vi "lv_icon.vi"(10 "Color icon in":T2, 11 "BW icon in":T2) -> (0 "Error code out":i32=43, 2 "Color icon out":T2, 3 "BW icon out":T2)   [LabVIEW 2020, in "lv_icon.lvlib"]
doc: "<p>Display this dialog box in one of the following ways:</p>\n\n<ul>\n<li>Double-click the <a href=\"nihelplauncher://docs/csh?context=lvcore_lvconcepts_using_icons\">icon</a> in the upper right corner of the front panel window, block diagram window, or <a href=\"nihelplauncher://docs/csh?context=lvcore_lvconcepts_custom_cont_ind_type\">Control Editor</a> window.</li>\n<li>Right-click the icon in the upper right corner of the front panel window, block diagram window, or <strong>Control Editor</strong> window and select <strong>Edit Icon</strong> from the shortcut menu.</li>\n<li>Select <strong>File<span class=\"U+187\">>></span>VI Properties</strong> or <strong>File<span class=\"U+187\">>></span>Control Properties</strong> to display the <a href=\"nihelplauncher://docs/csh?context=lvcore_lvdialog_vi_properties_dialog_box\">VI Properties</a> dialog box or <strong>Control Properties</strong> dialog box, respectively. Then select <strong>General</strong> from the <strong>Category</strong> pull-down menu and click the <strong>Edit Icon</strong> button.</li>\n<li>Right-click a project library, statechart, class, or XControl item in the <a href=\"nihelplauncher://docs/csh?context=lvcore_lvconcepts_using_labview_projects\">Project Explorer</a> window and select <strong> Properties</strong> from the shortcut menu to display the corresponding <strong>Properties</strong> dialog box. Then click the <strong>Edit</strong> button on the <strong>General Settings</strong> page.</li>\n</ul>\n\n<p>Use this dialog box to <a href=\"nihelplauncher://docs/csh?context=lvcore_lvhowto_creating_icons\">create and edit icons</a>.</p>"
uses:
  lv_icon.lvlib
  NIIconEditor/Class/Ants/Ants.lvclass
  NIIconEditor/Class/FakedArray/FakedArray.lvclass
  vi.lib/LabVIEW Icon API/lv_icon/Classes/Icon/Icon.lvclass
  NIIconEditor/Class/Icon Library/Glyph.lvclass
  vi.lib/LabVIEW Icon API/lv_icon/Controls/Pathes.ctl
  NIIconEditor/History/History.lvclass
  <vilib>/Utility/miscctls.llb/LVPoint32TypeDef.ctl
  NIIconEditor/Controls/Tools.ctl
  NIIconEditor/Controls/References Cluster.ctl
  NIIconEditor/Controls/Path&Icon.ctl
  vi.lib/LabVIEW Icon API/lv_icon/Controls/Graphic.ctl
  NIIconEditor/Global Variables/Data.vi
  <vilib>/Utility/miscctls.llb/LVMenuShortCut.ctl
  <resource>/plugins/IconEditor/Icon Editor Invoker Type.ctl
  NIIconEditor/Controls/Circle.ctl
  NIIconEditor/Controls/Dropper.ctl
  NIIconEditor/Controls/FCircle.ctl
  NIIconEditor/Controls/Fill.ctl
  NIIconEditor/Controls/FRect.ctl
  NIIconEditor/Controls/Line.ctl
  NIIconEditor/Controls/Move.ctl
  NIIconEditor/Controls/Pen.ctl
  NIIconEditor/Controls/Rubber.ctl
  NIIconEditor/Controls/Selection.ctl
  NIIconEditor/Controls/Text.ctl
  NIIconEditor/Controls/Rotate.ctl
  NIIconEditor/Controls/Flip.ctl
  vi.lib/LabVIEW Icon API/lv_icon/Controls/IEColor.ctl
  NIIconEditor/Controls/ColorChange.ctl
  NIIconEditor/Controls/Framework Templates.ctl
  NIIconEditor/Controls/TextMarker.ctl
  <vilib>/picture/picture.llb/imagedata.ctl
  vi.lib/LabVIEW Icon API/lv_icon/Controls/BodyText.ctl
  vi.lib/LabVIEW Icon API/lv_icon/Controls/Layer.ctl
  vi.lib/LabVIEW Icon API/lv_icon/Controls/Font.ctl
  NIIconEditor/Controls/LayerList.ctl
  vi.lib/LabVIEW Icon API/lv_icon/Controls/Alignment.ctl
  NIIconEditor/Controls/Arrow Up.ctl
  NIIconEditor/Controls/Arrow Down.ctl
  NIIconEditor/Controls/DeleteLayer.ctl
  NIIconEditor/Controls/NewLayer.ctl
  NIIconEditor/Controls/IERect.ctl
  NIIconEditor/Controls/Refresh.ctl
panel:
  out "LabVIEW Icon out":string
  in  "LabVIEW Icon in":string
  out "Terminals":picture
  out "Preview2":picture
  out "TextMarker":T1="^"
  in  "Help":bool
  in  "Cancel":bool
  in  "OK":bool
  out "XYZ":string="X: 14\nY: 31\nZ: 1"
  out "RGB":string="R: 0\nG: 0\nB: 0"
  out "Icon":picture
  out "Clipboard":picture
  in  "Tab Control":T3(tab)
  in  "refreshTemplates":T4
  out "templates path str":string
  in  "Templates":string(tree)="<All>"
  in  "Filter templates by keyword":string
  in  "Framework Templates":T5={"Scrollbar"=0, "Path & Icon 1"={"Rectangle"={"left"=0, "top"=0, "right"=32, "bottom"=32}, "Path"=path "C:/Users/tsandris/Documents/LabVIEW Data/Icon Templates/VI/Frameworks/_blank.png", "Image"=bytes[0], "Filter"="VI\\Frameworks", "FileName"="_blank"}, "Path & Icon 2"={"Rectangle"={"left"=0, "top"=0, "right"=32, "bottom"=32}, "Path"=path "C:/Users/tsandris/Documents/LabVIEW Data/Icon Templates/Library/Frameworks/_blank.png", "Image"=bytes[0], "Filter"="Library\\Frameworks", "FileName"="_blank"}, "Path & Icon 3"={"Rectangle"={"left"=0, "top"=0, "right"=0, "bottom"=0}, "Path"=path "", "Image"=bytes[0], "Filter"="", "FileName"=""}, "Path & Icon 4"={"Rectangle"={"left"=0, "top"=0, "right"=0, "bottom"=0}, "Path"=path "", "Image"=bytes[0], "Filter"="", "FileName"=""}, "Path & Icon 5"={"Rectangle"={"left"=0, "top"=0, "right"=0, "bottom"=0}, "Path"=path "", "Image"=bytes[0], "Filter"="", "FileName"=""}, "Path & Icon 6"={"Rectangle"={"left"=0, "top"=0, "right"=0, "bottom"=0}, "Path"=path "", "Image"=bytes[0], "Filter"="", "FileName"=""}, "Path & Icon 7"={"Rectangle"={"left"=0, "top"=0, "right"=0, "bottom"=0}, "Path"=path "", "Image"=bytes[0], "Filter"="", "FileName"=""}, "Path & Icon 8"={"Rectangle"={"left"=0, "top"=0, "right"=0, "bottom"=0}, "Path"=path "", "Image"=bytes[0], "Filter"="", "FileName"=""}, "Path & Icon 9"={"Rectangle"={"left"=0, "top"=0, "right"=0, "bottom"=0}, "Path"=path "", "Image"=bytes[0], "Filter"="", "FileName"=""}, "Path & Icon 10"={"Rectangle"={"left"=0, "top"=0, "right"=0, "bottom"=0}, "Path"=path "", "Image"=bytes[0], "Filter"="", "FileName"=""}, "Path & Icon 11"={"Rectangle"={"left"=0, "top"=0, "right"=0, "bottom"=0}, "Path"=path "", "Image"=bytes[0], "Filter"="", "FileName"=""}, "Path & Icon 12"={"Rectangle"={"left"=0, "top"=0, "right"=0, "bottom"=0}, "Path"=path "", "Image"=bytes[0], "Filter"="", "FileName"=""}, "Path & Icon 13"={"Rectangle"={"left"=0, "top"=0, "right"=0, "bottom"=0}, "Path"=path "", "Image"=bytes[0], "Filter"="", "FileName"=""}, "Path & Icon 14"={"Rectangle"={"left"=0, "top"=0, "right"=0, "bottom"=0}, "Path"=path "", "Image"=bytes[0], "Filter"="", "FileName"=""}, "Path & Icon 15"={"Rectangle"={"left"=0, "top"=0, "right"=0, "bottom"=0}, "Path"=path "", "Image"=bytes[0], "Filter"="", "FileName"=""}, "Path & Icon 16"={"Rectangle"={"left"=0, "top"=0, "right"=0, "bottom"=0}, "Path"=path "", "Image"=bytes[0], "Filter"="", "FileName"=""}, "Path & Icon 17"={"Rectangle"={"left"=0, "top"=0, "right"=0, "bottom"=0}, "Path"=path "", "Image"=bytes[0], "Filter"="", "FileName"=""}, "Path & Icon 18"={"Rectangle"={"left"=0, "top"=0, "right"=0, "bottom"=0}, "Path"=path "", "Image"=bytes[0], "Filter"="", "FileName"=""}, "Path & Icon 19"={"Rectangle"={"left"=0, "top"=0, "right"=0, "bottom"=0}, "Path"=path "", "Image"=bytes[0], "Filter"="", "FileName"=""}, "Path & Icon 20"={"Rectangle"={"left"=0, "top"=0, "right"=0, "bottom"=0}, "Path"=path "", "Image"=bytes[0], "Filter"="", "FileName"=""}, "Path & Icon 21"={"Rectangle"={"left"=0, "top"=0, "right"=0, "bottom"=0}, "Path"=path "", "Image"=bytes[0], "Filter"="", "FileName"=""}, "Path & Icon 22"={"Rectangle"={"left"=0, "top"=0, "right"=0, "bottom"=0}, "Path"=path "", "Image"=bytes[0], "Filter"="", "FileName"=""}, "Path & Icon 23"={"Rectangle"={"left"=0, "top"=0, "right"=0, "bottom"=0}, "Path"=path "", "Image"=bytes[0], "Filter"="", "FileName"=""}, "Path & Icon 24"={"Rectangle"={"left"=0, "top"=0, "right"=0, "bottom"=0}, "Path"=path "", "Image"=bytes[0], "Filter"="", "FileName"=""}, "Path & Icon 25"={"Rectangle"={"left"=0, "top"=0, "right"=0, "bottom"=0}, "Path"=path "", "Image"=bytes[0], "Filter"="", "FileName"=""}, "Path & Icon 26"={"Rectangle"={"left"=0, "top"=0, "right"=0, "bottom"=0}, "Path"=path "", "Image"=bytes[0], "Filter"="", "FileName"=""}, "Path & Icon 27"={"Rectangle"={"left"=0, "top"=0, "right"=0, "bottom"=0}, "Path"=path "", "Image"=bytes[0], "Filter"="", "FileName"=""}, "Path & Icon 28"={"Rectangle"={"left"=0, "top"=0, "right"=0, "bottom"=0}, "Path"=path "", "Image"=bytes[0], "Filter"="", "FileName"=""}, "Path & Icon 29"={"Rectangle"={"left"=0, "top"=0, "right"=0, "bottom"=0}, "Path"=path "", "Image"=bytes[0], "Filter"="", "FileName"=""}, "Path & Icon 30"={"Rectangle"={"left"=0, "top"=0, "right"=0, "bottom"=0}, "Path"=path "", "Image"=bytes[0], "Filter"="", "FileName"=""}}
  in  "Body Text":T7={"Line 1 text"="", "Line 2 text"="", "Line 3 text"="", "Line 4 text"="", "Line 1 color"=0, "Line 2 color"=0, "Line 3 color"=0, "Line 4 color"=0, "Body Text Spec"={"Font"="", "Alignment"=1, "Size"=9}, "Center text vertically"=TRUE, "Capitalize Text"=TRUE} {"Body Text Spec"."Alignment" items=["left", "center", "right"]}
  in  "Filter glyphs by keyword":string
  in  "Glyphs":string(tree)="<All>"
  out "glyph path str":string
  out "Glyphs []":T6[][](array[typedef])
  in  "refreshGlyphs":T4
  in  "Add Layer":T10
  in  "Remove Layer":T11
  in  "Move Down":T12
  in  "Move Up":T13
  in  "Icon Template":T14={"LayerIcon"=bytes[0], "LayerName"="", "Opacity"=100, "Visibility?"=TRUE} {"Opacity" scale=0.0..100.0}
  in  "Icon Text":T14={"LayerIcon"=bytes[0], "LayerName"="Icon Text", "Opacity"=100, "Visibility?"=TRUE} {"Opacity" scale=0.0..100.0}
  in  "User Layers":T15={"Scrollbar"=0, "Layer 1"={"LayerIcon"=bytes[0], "LayerName"="VI Icon", "Opacity"=100, "Visibility?"=TRUE}, "Layer 2"={"LayerIcon"=bytes[3230], "LayerName"="", "Opacity"=100, "Visibility?"=TRUE}, "Layer 3"={"LayerIcon"=bytes[3230], "LayerName"="", "Opacity"=100, "Visibility?"=TRUE}, "Layer 4"={"LayerIcon"=bytes[3230], "LayerName"="", "Opacity"=100, "Visibility?"=TRUE}} {"Layer 4"."Opacity" scale=0.0..100.0; "Layer 3"."Opacity" scale=0.0..100.0; "Layer 2"."Opacity" scale=0.0..100.0; "Layer 1"."Opacity" scale=0.0..100.0}
  out "Preview":picture
  in  "Horizontal Flip":T16
  in  "Clockwise Rotate":T17
  in  "Swap":T18
  in  "Line Color":T19
  in  "Fill Color":T19=16777215
  in  "Tools":T20=enum."Rectangle"
  # "Clipboard control. Anything made on this\ncontrol will show up in the clipboard image data."
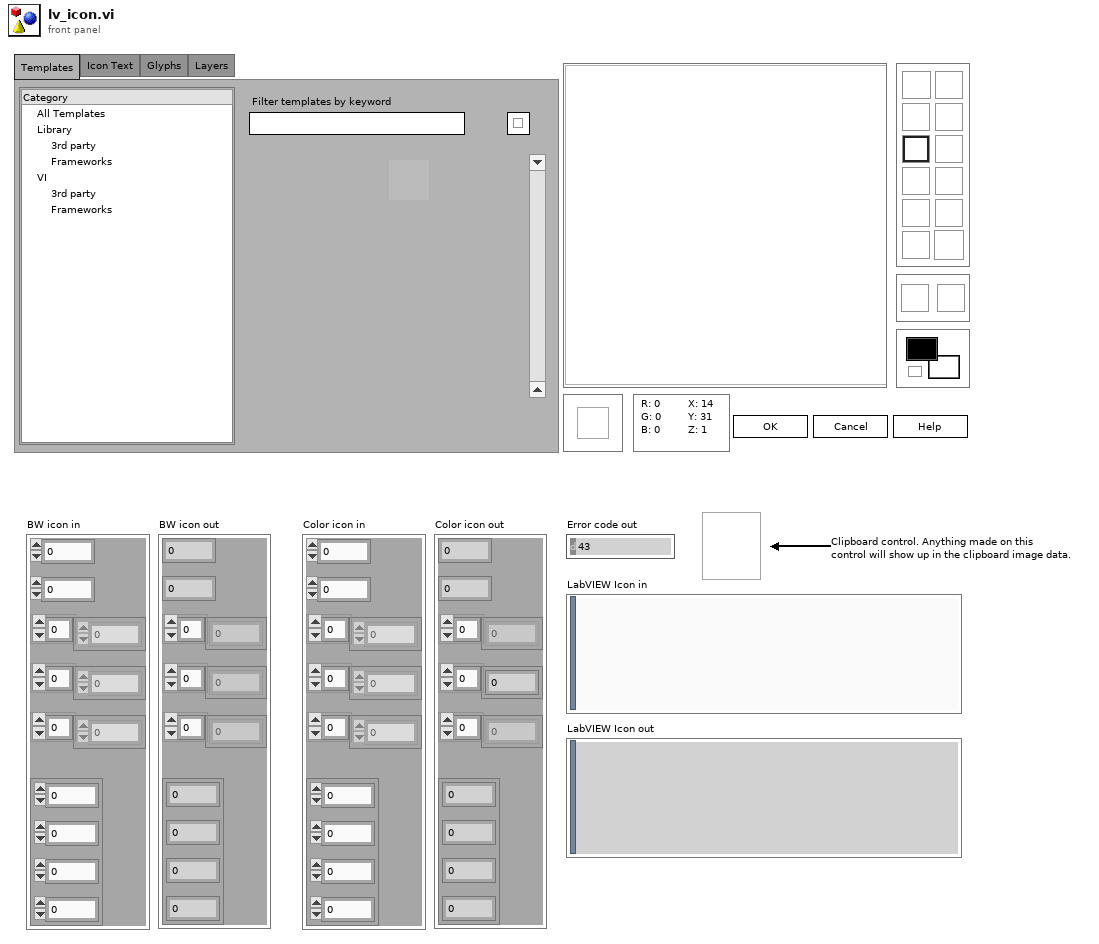
[diagram p1: front panel]
types:
  T1 = typedef "TextMarker.ctl" = string
  T2 = typedef "imagedata.ctl" = cluster{"image type":i32, "image depth":i32, "image":u8[], "mask":u8[], "colors":u32[], "Rectangle":cluster{"left":i16, "top":i16, "right":i16, "bottom":i16}}
  T3 = enum32{"Templates", "Icon Text", "Glyphs", "Layers"}
  T4 = typedef "Refresh.ctl" = bool
  T5 = typedef "Framework Templates.ctl" = cluster{"Scrollbar":i32, "Path & Icon 1":T6, "Path & Icon 2":T6, "Path & Icon 3":T6, "Path & Icon 4":T6, "Path & Icon 5":T6, "Path & Icon 6":T6, "Path & Icon 7":T6, "Path & Icon 8":T6, "Path & Icon 9":T6, "Path & Icon 10":T6, "Path & Icon 11":T6, "Path & Icon 12":T6, "Path & Icon 13":T6, "Path & Icon 14":T6, "Path & Icon 15":T6, "Path & Icon 16":T6, "Path & Icon 17":T6, "Path & Icon 18":T6, "Path & Icon 19":T6, "Path & Icon 20":T6, "Path & Icon 21":T6, "Path & Icon 22":T6, "Path & Icon 23":T6, "Path & Icon 24":T6, "Path & Icon 25":T6, "Path & Icon 26":T6, "Path & Icon 27":T6, "Path & Icon 28":T6, "Path & Icon 29":T6, "Path & Icon 30":T6}
  T6 = typedef "Graphic.ctl" = cluster{"Rectangle":cluster{"left":i16, "top":i16, "right":i16, "bottom":i16}, "Path":path, "Image":picture, "Filter":string, "FileName":string}
  T7 = typedef "BodyText.ctl" = cluster{"Line 1 text":string, "Line 2 text":string, "Line 3 text":string, "Line 4 text":string, "Line 1 color":u32, "Line 2 color":u32, "Line 3 color":u32, "Line 4 color":u32, "Body Text Spec":cluster{"Font":T8, "Alignment":T9, "Size":u8}, "Center text vertically":bool, "Capitalize Text":bool}
  T8 = typedef "Font.ctl" = string
  T9 = typedef "Alignment.ctl" = u16
  T10 = typedef "NewLayer.ctl" = bool
  T11 = typedef "DeleteLayer.ctl" = bool
  T12 = typedef "Arrow Down.ctl" = bool
  T13 = typedef "Arrow Up.ctl" = bool
  T14 = typedef "Layer.ctl" = cluster{"LayerIcon":picture, "LayerName":string, "Opacity":u8, "Visibility?":bool}
  T15 = typedef "LayerList.ctl" = cluster{"Scrollbar":i32, "Layer 1":T14, "Layer 2":T14, "Layer 3":T14, "Layer 4":T14}
  T16 = typedef "Flip.ctl" = bool
  T17 = typedef "Rotate.ctl" = bool
  T18 = typedef "ColorChange.ctl" = bool
  T19 = typedef "IEColor.ctl" = u32
  T20 = typedef "Tools.ctl" = enum32{"Pencil", "Line", "Dropper", "Fill", "Rectangle", "Filled Rectangle", "Ellipse", "Filled Ellipse", "Eraser", "Text", "Select", "Move"}
  T21 = typedef "Icon Editor Invoker Type.ctl" = enum32{"Unknown Icon Source", "VI Icon", "Library Icon (any library type)", "Palette icon", "Icon from App Method"}
  T22 = enum32{"Invalid", "Default", "Floating", "Floating/Auto-Hide", "Modal"}
  T23 = enum32{"Invalid", "Standard", "Closed", "Hidden", "Minimized", "Maximized"}
  T24 = typedef "lv_icon.lvlib/References Cluster.ctl" = cluster{"Add Layer":refnum<vi>, "Remove Layer":refnum<vi>, "Line Text":refnum<vi>[], "Body Text Spec":refnum<vi>, "DNL_Font":refnum<vi>, "glyph path str":refnum<vi>, "templates path str":refnum<vi>, "Arrow Up":refnum<vi>, "Arrow Down":refnum<vi>, "IE VI Ref":refnum<vi>, "Glyphs tree":refnum<vi>, "Templates tree":refnum<vi>, "Layer Icon Text":refnum<vi>, "Layer Template":refnum<vi>, "Body Text":refnum<vi>, "Search Templates":refnum<vi>, "TextMarker":refnum<vi>, "Tab Control":refnum<vi>, "Search Glyphs":refnum<vi>, "Line Color":refnum<vi>, "DNL_Glyphs []":refnum<vi>, "Fill Color":refnum<vi>, "Tools":refnum<vi>, "Icon":refnum<vi>, "Preview":refnum<vi>, "Ants":refnum<vi>, "Terminals":refnum<vi>, "menu reference":refnum<k9>, "LayerNames":refnum<vi>[], "GlyphLoadAnimation":refnum<vi>, "TemplateLoadAnimation":refnum<vi>, "refreshGlyphs":refnum<vi>, "refreshTemplates":refnum<vi>}
  T25 = typedef "Who Invoked Icon Editor.ctl" = cluster{"Icon Editor Invoker Type":T21, "App Refnum of Invoker":refnum<vi>, "Qualified Name of Invoker":string, "Path to Invoker":path}
  T26 = typedef "LVMenuShortCut.ctl" = cluster{"Include Shift Key?":bool, "Include Ctrl Key?":bool, "Shortcut Key":string}
  T27 = cluster{"Global stop?":refnum<user-event>, "Templates":refnum<user-event>, "Glyphs":refnum<user-event>}
  T28 = typedef "lv_icon.lvlib/Global Data.ctl" = cluster{"Class":T29, "Ref":T24, "Support":T30}
  T29 = typedef "IE Classes.ctl" = cluster{"Ants":refnum<class "Ants.lvclass">, "Layer":refnum<class "FakedArray.lvclass">, "Templates":refnum<class "FakedArray.lvclass">, "Icon":refnum<class "Icon.lvclass">, "Glyph":refnum<class "Glyph.lvclass">, "Settings":refnum<class "Settings.lvclass">, "Tools":refnum<class "Tools Paint.lvclass">}
  T30 = typedef "SupportClass.ctl" = cluster{"AntsRect":cluster{"left":i16, "top":i16, "right":i16, "bottom":i16}, "Mouse Move Coords":T31, "Mouse Down Coords":T31, "Temp Coord":T31, "Action":T32, "Edge Color":T19, "Fill Color":T19, "Mouse Down?":bool, "Draft Mode?":bool, "Temp Icon":picture, "CTRL Pressed":bool, "Move Selection?":bool, "AntsRect Orig":cluster{"left":i16, "top":i16, "right":i16, "bottom":i16}, "Text":string, "TM Set?":bool, "Mouse inside icon?":bool, "Tool (old value)":u32, "Pencil Move Color":u32, "Swap Colors?":bool, "Shift pressed?":bool}
  T31 = typedef "LVPoint32TypeDef.ctl" = cluster{"Horizontal":i32, "Vertical":i32}
  T32 = typedef "SupportClass_Action.ctl" = enum16{"Default", "Move Selection", "Glyph Library", "Tool"}
  T33 = typedef "Pathes.ctl" = enum16{"Root Path", "Icon Templates", "Icon Templates VI", "Icon Templates Lib", "Glyphs"}
  T34 = typedef "Path&Icon.ctl" = cluster{"Rectangle":cluster{"left":i16, "top":i16, "right":i16, "bottom":i16}, "Path":path, "Image":picture, "Filter":string, "FileName":string}
  T35 = typedef "lveventtype.ctl" = enum32{"Null", "Timeout", "Annotation Menu Selection", "Annotation Menu Selection?", "App Instance Close", "App Instance Close?", "Autoscale Range Change", "Bookmark Info Change", "Cell Edit", "Cell Edit?", "Cursor Grab", "Cursor Grab?", "Cursor Menu Selection", "Cursor Menu Selection?", "Cursor Move", "Cursor Release", "Data Change", "Direction Change", "Display State Change", "Drag Ended", "Drag Enter", "Drag Leave", "Drag Over", "Drag Source Update", "Drag Starting", "Drag Starting?", "Drop", "Exec State Change", "Key Down", "Key Down?", "Key Repeat", "Key Repeat?", "Key Up", "Listbox Double Click", "Menu Activation?", "Menu Selection (App)", "Menu Selection? (App)", "Menu Selection (User)", "Mouse Down", "Mouse Down?", "Mouse Enter", "Mouse Leave", "Mouse Move", "Mouse Up", "Mouse Wheel", "NI Security User Change (App)", "Pane Size", "Panel Close", "Panel Close?", "Panel Resize", "Plot Attribute Change", "Scale Range Change", "Shortcut Menu Activation?", "Shortcut Menu Selection (App)", "Shortcut Menu Selection? (App)", "Shortcut Menu Selection (User)", "Tree Double Click", "Tree Drag", "Tree Drag?", "Tree Drop", "Tree Drop?", "Tree Item Close", "Tree Item Close?", "Tree Item Open", "Tree Item Open?", "URL Change?", "User Event", "Value Change"}
  T36 = typedef "eventvkey.ctl" = enum16{"ASCII", "Enter", "Return", "Shift", "Ctrl", "Alt", "Cmd", "Opt", "Caps", "NumLock", "Clear", "Break", "Up", "Down", "Left", "Right", "Insert", "Delete", "Home", "End", "PageUp", "PageDown", "Escape", "Help", "Pause", "ScrollLock", "F1", "F2", "F3", "F4", "F5", "F6", "F7", "F8", "F9", "F10", "F11", "F12", "F13", "F14", "F15", "F16", "F17", "F18", "F19", "F20", "F21", "F22", "F23", "F24", "Play", "VolumeUp", "VolumeDown", "Mute", "Two Byte Char"}
  T37 = cluster{"Shift":bool, "Ctrl":bool, "Alt":bool, "Cmd":bool, "Opt":bool}
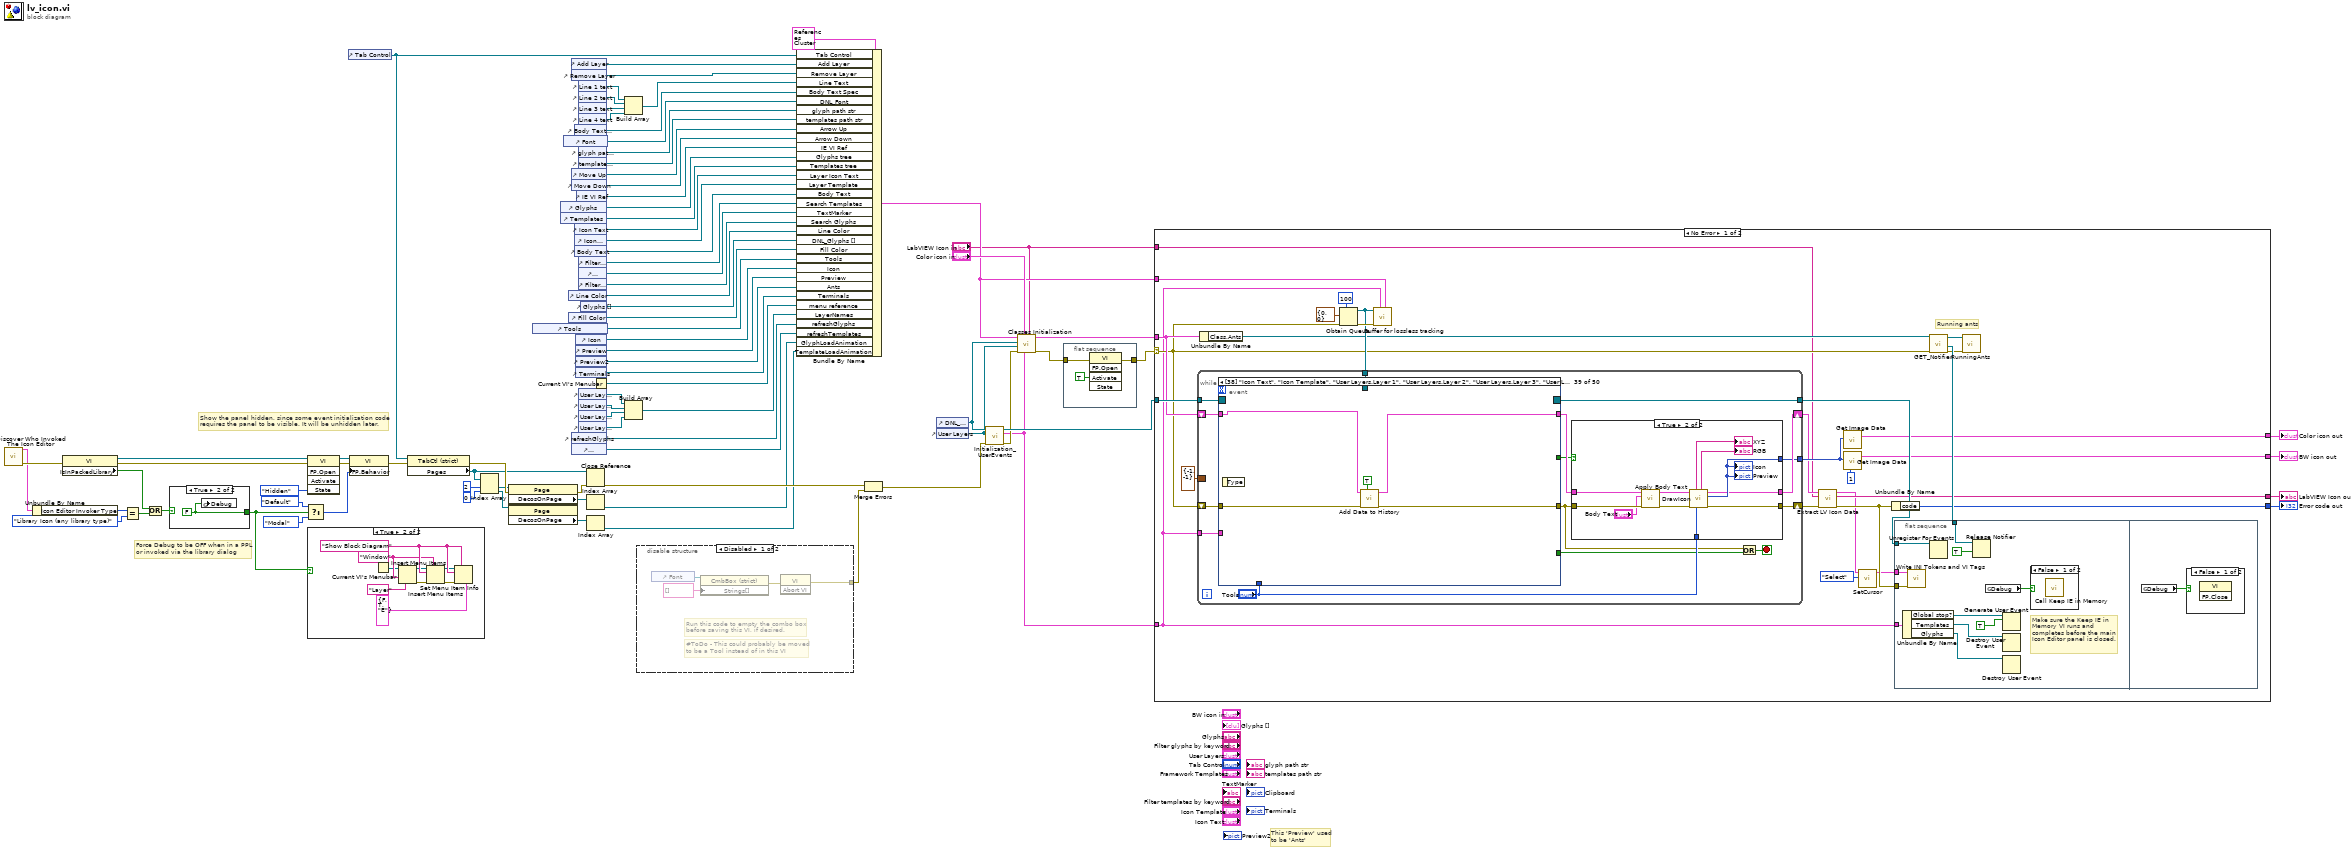
[diagram p0: block diagram]
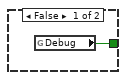
[diagram p2: hidden frame]
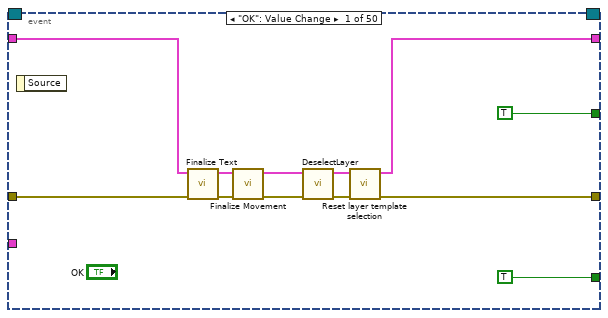
[diagram p6: hidden frame]
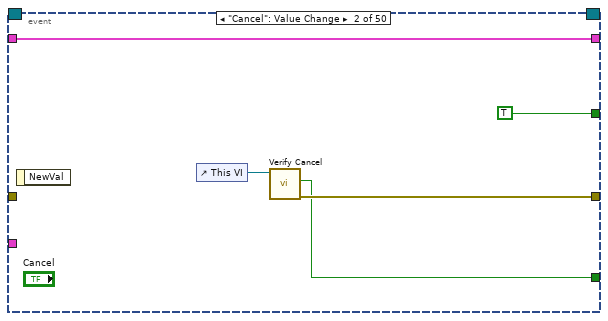
[diagram p7: hidden frame]
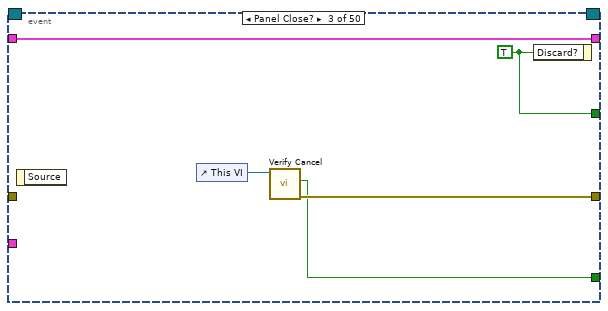
[diagram p8: hidden frame]
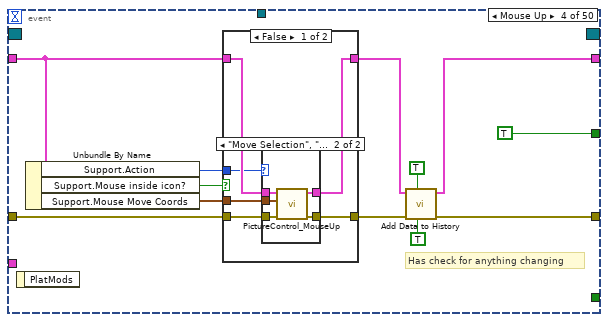
[diagram p9: hidden frame]
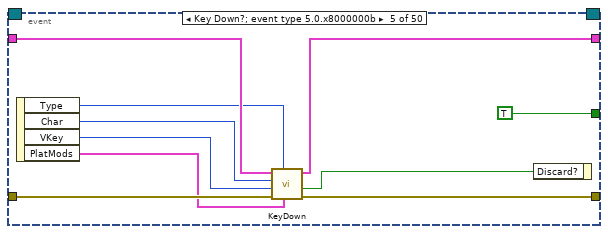
[diagram p12: hidden frame]
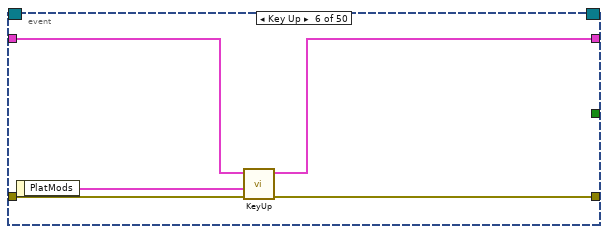
[diagram p13: hidden frame]
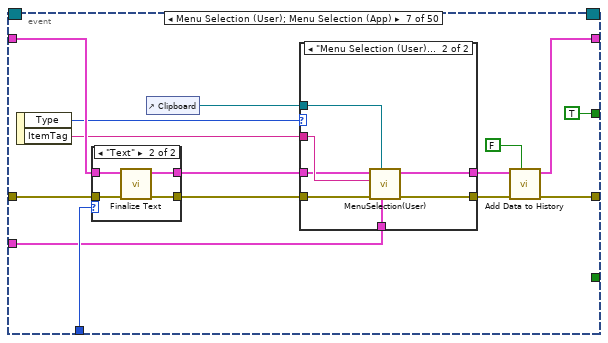
[diagram p14: hidden frame]
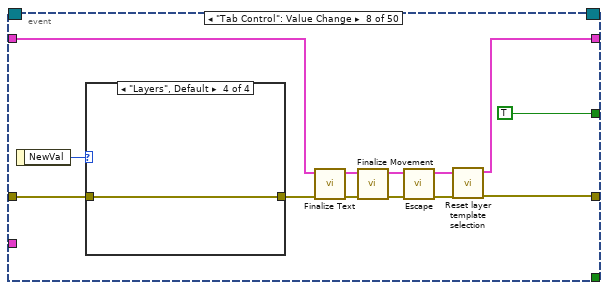
[diagram p17: hidden frame]
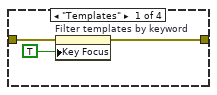
[diagram p18: hidden frame]
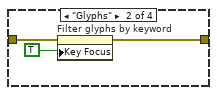
[diagram p19: hidden frame]
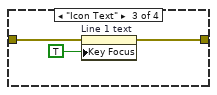
[diagram p20: hidden frame]
diagram:
  # "Force Debug to be OFF when in a PPL\nor invoked via the library dialog"
  # "Show the panel hidden, since some event initialization code requires the panel to be visible. It will be unhidden later."
  # "This 'Preview' used\nto be 'Ants'"
  n1 = call <resource>:"Discover Who Invoked The Icon Editor.vi"() -> ("error out"=w7:errorcluster, "Who Invoked The Icon Editor?"=w6:T25)  [unwired: 10 in]
  n2 = Unbundle By Name(w6) -> ("Icon Editor Invoker Type"=w5:T21)
  n3 = property class="VI"(error in=w7) -> (reference out=w9:refnum<vi>, error out=w8:errorcluster, "IsInPackedLibrary"=w2:bool)  [unwired: 1 in]
  n4 = Equal?(x=w5, y=Icon_Editor_Invoker_Type."Library Icon (any library type)") -> (x = y?=w3:bool)
  n5 = Or(x=w2, y=w3) -> (x .or. y?=w1:bool)
  n6 = case shown="True" w1 {
    tunnel: [w87 w88] -> w10
    frame False {
      n7 = global read "Data.vi" "Debug"() -> (w87:bool)
    }
    frame True {
      w88 = FALSE
      n8 = global write "Data.vi" "Debug"(w88) -> ()
    }
  }
  n9 = Select(t=T22."Default" ("Front Panel Window:Behavior"), s=w10, f=T22."Modal" ("Front Panel Window:Behavior")) -> (s? t:f=w11:T22)
  n10 = invoke class="VI" method="FP.Open"(reference=w9, error in=w8, "State"=T23."Hidden") -> (reference out=w14:refnum<vi>, error out=w16:errorcluster)  [unwired: 2 in, 3 out]
  n11 = case shown="True" w10 {
    frame False {
    }
    frame True {
      w97 = "Show Block Diagram"
      w92 = "Window" ("menu tag")
      n12 = Current VI's Menubar() -> (w89:refnum<k9>)
      n13 = Insert Menu Items(4:"Layer" ("after item"), 7:w92, 9:w89) -> (0:w94:errorcluster, 3:w95:refnum<k9>)  [unwired: 3 in, 1 out]
      n14 = Insert Menu Items(5:w92, 6:w94, 8:w97, 9:w95) -> (0:w90:errorcluster, 3:w91:refnum<k9>)  [unwired: 2 in, 1 out]
      n15 = Set Menu Item Info(4:T26 {"Include Shift Key?"=FALSE, "Include Ctrl Key?"=TRUE, "Shortcut Key"="E"} ("short cut"), 7:w97, 8:w90, 10:w97, 11:w91) -> ()  [unwired: 2 in, 2 out]
    }
  }
  n16 = control-ref of="Tab Control"() -> (w19:refnum<vi>)
  n17 = property class="VI"(reference=w14, error in=w16, "FP.Behavior"=w11) -> (error out=w15:errorcluster)  [unwired: 1 out]
  n18 = property class="TabCtl (strict)"(reference=w19, error in=w15) -> (error out=w29:errorcluster, "Pages"=w21:refnum<vi>[])  [unwired: 1 out]
  n19 = Index Array(array=w21, index #1=2 ("index"), index #2=0 ("index")) -> (element #1=w25:refnum<vi>, element #2=w26:refnum<vi>)
  n20 = property class="Page"(reference=w25, error in=w29) -> (error out=w22:errorcluster, "DecosOnPage"=w24:refnum<vi>[])  [unwired: 1 out]
  n21 = property class="Page"(reference=w26) -> ("DecosOnPage"=w23:refnum<vi>[])  [unwired: 1 in, 2 out]
  n22 = control-ref of="Tools"() -> (w83:refnum<vi>)
  n23 = control-ref of="Glyphs"() -> (w67:refnum<vi>)
  n24 = control-ref of="Templates"() -> (w68:refnum<vi>)
  n25 = control-ref of="Font"() -> (w49:refnum<vi>)
  n26 = control-ref of="Line Color"() -> (w81:refnum<vi>)
  n27 = control-ref of="Fill Color"() -> (w82:refnum<vi>)
  n28 = control-ref of="Add Layer"() -> (w52:refnum<vi>)
  n29 = control-ref of="Remove Layer"() -> (w53:refnum<vi>)
  n30 = control-ref of="Move Up"() -> (w64:refnum<vi>)
  n31 = control-ref of="Move Down"() -> (w65:refnum<vi>)
  n32 = control-ref of="refreshGlyphs"() -> (w39:refnum<vi>)
  n33 = control-ref of="refreshTemplates"() -> (w40:refnum<vi>)
  n34 = control-ref of="Body Text Spec"() -> (w61:refnum<vi>)
  n35 = control-ref of="Icon Text"() -> (w70:refnum<vi>)
  n36 = control-ref of="Icon Template"() -> (w71:refnum<vi>)
  n37 = control-ref of="Body Text"() -> (w76:refnum<vi>)
  n38 = control-ref of="Icon"() -> (w84:refnum<vi>)
  n39 = control-ref of="Preview"() -> (w85:refnum<vi>)
  n40 = control-ref of="Preview2"() -> (w60:refnum<vi>)
  n41 = control-ref of="Terminals"() -> (w75:refnum<vi>)
  n42 = control-ref of="IE VI Ref"() -> (w66:refnum<vi>)
  n43 = control-ref of="Line 1 text"() -> (w55:refnum<vi>)
  n44 = control-ref of="Line 2 text"() -> (w56:refnum<vi>)
  n45 = control-ref of="Line 3 text"() -> (w57:refnum<vi>)
  n46 = control-ref of="Line 4 text"() -> (w58:refnum<vi>)
  n47 = control-ref of="glyph path str"() -> (w62:refnum<vi>)
  n48 = control-ref of="templates path str"() -> (w63:refnum<vi>)
  n49 = control-ref of="Filter templates by keyword"() -> (w78:refnum<vi>)
  n50 = control-ref of="TextMarker"() -> (w79:refnum<vi>)
  n51 = control-ref of="Filter glyphs by keyword"() -> (w80:refnum<vi>)
  n52 = control-ref of="User Layer 1"() -> (w44:refnum<vi>)
  n53 = control-ref of="User Layer 2"() -> (w45:refnum<vi>)
  n54 = control-ref of="User Layer 3"() -> (w46:refnum<vi>)
  n55 = control-ref of="User Layer 4"() -> (w47:refnum<vi>)
  n56 = control-ref of="Glyphs []"() -> (w50:refnum<vi>)
  n57 = Close Reference(reference=w21, error in (no error)=w22) -> (error out=w20:errorcluster)
  n58 = Index Array(array=w24) -> (element=w18:refnum<vi>)  [unwired: 1 in]
  n59 = Index Array(array=w23) -> (element=w17:refnum<vi>)  [unwired: 1 in]
  n60 = Current VI's Menubar() -> (w74:refnum<k9>)
  n61 = Build Array(w55, w56, w57, w58) -> (w54:refnum<vi>[])
  n62 = Build Array(w44, w45, w46, w47) -> (w42:refnum<vi>[])
  n63 = disable-structure shown="Disabled" {
    disable-tunnel: [w98 _] -> w31
    frame Disabled {
      # "#ToDo - This could probably be moved\nto be a Tool instead of in this VI"
      # "Run this code to empty the combo box\nbefore saving this VI, if desired."
      n64 = control-ref of="Font"() -> (w101:refnum<vi>)
      n65 = property class="CmbBox (strict)"(reference=w101, "Strings[]"=string[] [] ("Strings []")) -> (error out=w99:errorcluster)  [unwired: 1 in, 1 out]
      n66 = invoke class="VI" method="Abort VI"(error in=w99) -> (error out=w98:errorcluster)  [unwired: 2 in, 2 out]
    }
    frame Enabled {
    }
  }
  n67 = Bundle By Name(cluster=T24 {"Add Layer"=refnum, "Remove Layer"=refnum, "Line Text"=[], "Body Text Spec"=refnum, "DNL_Font"=refnum, "glyph path str"=refnum, "templates path str"=refnum, "Arrow Up"=refnum, "Arrow Down"=refnum, "IE VI Ref"=refnum, "Glyphs tree"=refnum, "Templates tree"=refnum, "Layer Icon Text"=refnum, "Layer Template"=refnum, "Body Text"=refnum, "Search Templates"=refnum, "TextMarker"=refnum, "Tab Control"=refnum, "Search Glyphs"=refnum, "Line Color"=refnum, "DNL_Glyphs []"=refnum, "Fill Color"=refnum, "Tools"=refnum, "Icon"=refnum, "Preview"=refnum, "Ants"=refnum, "Terminals"=refnum, "menu reference"=refnum, "LayerNames"=[], "GlyphLoadAnimation"=refnum, "TemplateLoadAnimation"=refnum, "refreshGlyphs"=refnum, "refreshTemplates"=refnum} ("references"), "Tab Control"=w19, "Add Layer"=w52, "Remove Layer"=w53, "Line Text"=w54, "Body Text Spec"=w61, "DNL_Font"=w49, "glyph path str"=w62, "templates path str"=w63, "Arrow Up"=w64, "Arrow Down"=w65, "IE VI Ref"=w66, "Glyphs tree"=w67, "Templates tree"=w68, "Layer Icon Text"=w70, "Layer Template"=w71, "Body Text"=w76, "Search Templates"=w78, "TextMarker"=w79, "Search Glyphs"=w80, "Line Color"=w81, "DNL_Glyphs []"=w50, "Fill Color"=w82, "Tools"=w83, "Icon"=w84, "Preview"=w85, "Ants"=w60, "Terminals"=w75, "menu reference"=w74, "LayerNames"=w42, "refreshGlyphs"=w39, "refreshTemplates"=w40, "GlyphLoadAnimation"=w18, "TemplateLoadAnimation"=w17) -> (w43:T24)
  n68 = Merge Errors(w20, w31) -> (w30:errorcluster)
  n69 = control-ref of="DNL_Framework Templates"() -> (w33:refnum<vi>)
  n70 = control-ref of="User Layers"() -> (w32:refnum<vi>)
  n71 = call "Initialization_UserEvents.vi"("error in"=w30, "Layer Clusters"=w32, "DNL_Framework Templates"=w33) -> ("error out"=w72:errorcluster, "User events"=w34:T27, "Events"=w77:refnum<event-registration>)  [unwired: 6 out]
  n72 = call "Classes Initialization.vi"("LabVIEW Icon in"="LabVIEW Icon in", "User events"=w34, "Color icon in"="Color icon in", "error in"=w72, "Layer Clusters"=w32, "DNL_Framework Templates"=w33, "Ref Cluster"=w43) -> ("error out"=w36:errorcluster, "Data out"=w59:T28)  [unwired: 3 out]
  n73 = flat-sequence {
    tunnel: w36 -> [w103]
    tunnel: [w102] -> w35
    frame #0 {
      n74 = invoke class="VI" method="FP.Open"(error in=w103, "Activate"=TRUE ("Activate?")) -> (error out=w102:errorcluster)  [unwired: 3 in, 4 out]
    }
  }
  n75 = case shown="No Error" w35 {
    selector: w35 -> [w114 w803]
    tunnel: w77 -> [w131 _]
    tunnel: [w129 w804] -> w73
    tunnel: [w126 _] -> w69
    tunnel: w34 -> [w105 _]
    tunnel: w59 -> [w119 _]
    tunnel: w43 -> [w117 _]
    tunnel: [w116 _] -> w51
    tunnel: "LabVIEW Icon in" -> [w109 w802]
    tunnel: [w112 w802] -> w48
    frame No Error {
      # "Running ants"
      n76 = Unbundle By Name(w119) -> ("Class.Ants"=w118:refnum<class "Ants.lvclass">)
      n77 = Obtain Queue(max queue size (-1, unlimited)=100, element data type=T31 {"Horizontal"=0, "Vertical"=0} ("Coords"), error in (no error)=w114) -> (queue out=w120:refnum<queue>, error out=w121:errorcluster)  [unwired: 1 in, 2 out]
      n78 = while {
        shift-right: [w137] -> w111
        shift-left: w114 -> [w144]
        tunnel: [w141] -> w132
        tunnel: w131 -> [w140]
        tunnel: [w139] -> w128
        tunnel: w120 -> [w135]
        shift-right: [w146] -> w113
        shift-left: w119 -> [w134]
        border: T31 {"Horizontal"=-1, "Vertical"=-1} ("Corrected Out") -> [_]
        tunnel: w105 -> [w133]
        stop <- w142 stop-if-true
        n79 = event shown="[38] \"Icon Text\", \"Icon Template\", \"User Layers.Layer 1\", \"User Layers.Layer 2\", \"User Layers.Layer 3\", \"User Layers.Layer 4\": Mouse Leave;  \"Icon Text\", \"Icon Template\", \"User Layers.Layer 4\", \"User Layers.Layer 3\", \"User Layers.Layer 2\", \"User Layers.Layer 1\": Mouse Up" {
          selector: w140 -> [_ _ _ _ _ _ _ _ _ _ _ _ _ _ _ _ _ _ _ _ _ _ _ _ _ _ _ _ _ _ _ _ _ _ _ _ _ _ _ _ _ _ _ _ _ _ _ _ _ _]
          dyn-events: [_ _ _ _ _ _ _ _ _ _ _ _ _ _ _ _ _ _ _ _ _ _ _ _ _ _ _ _ _ _ _ _ _ _ _ _ _ _ _ _ _ _ _ _ _ _ _ _ _ _] -> w141
          timeout: _ -> [_ _ _ _ _ _ _ _ _ _ _ _ _ _ _ _ _ _ _ _ _ _ _ _ _ _ _ _ _ _ _ _ _ _ _ _ _ _ _ _ _ _ _ _ _ _ _ _ _ _]
          tunnel: [w166 w176 w181 w186 w218 w224 w228 w263 w284 w294 w307 w324 w328 w334 w338 w351 w363 w377 w392 w403 w428 w435 w446 w462 w483 w491 w509 w529 w534 w538 w545 w556 w571 w586 w601 w612 w625 w641 w650 w660 w682 w695 w710 w720 w722 w741 w758 w778 w785 w787] -> w138
          tunnel: w144 -> [w168 _ _ w192 w219 w223 w236 w265 w285 w295 w307 w325 w331 w336 w343 w355 w362 w371 w394 w412 w429 w438 w451 w464 w486 w505 w517 w530 w535 w539 w546 w563 w576 w589 w605 w613 w631 w645 w651 w662 w685 w703 w713 w719 w731 w748 w762 w779 w785 w788]
          tunnel: [TRUE w175 w180 _ _ _ _ _ _ _ _ _ _ _ _ _ _ _ _ _ _ _ _ _ _ _ _ _ _ _ _ _ _ _ _ _ _ _ _ _ _ _ _ _ _ _ _ _ _ _] -> w143
          tunnel: "Tools" -> [_ _ _ _ _ _ w234 _ w283 _ _ _ _ _ _ _ _ _ _ _ _ _ _ _ _ _ _ _ _ _ _ _ _ _ _ _ _ _ _ _ _ _ _ _ _ _ _ _ _ _]
          tunnel: [TRUE TRUE ("Yes") w179 TRUE ("Yes") TRUE _ TRUE TRUE TRUE TRUE _ TRUE TRUE _ TRUE TRUE TRUE TRUE TRUE TRUE _ _ TRUE TRUE _ _ _ _ _ _ TRUE TRUE TRUE _ TRUE _ TRUE _ _ TRUE TRUE _ _ _ _ _ TRUE _ _ _] -> w136
          tunnel: w135 -> [_ _ _ _ _ _ _ _ _ w292 _ _ _ _ _ _ _ _ _ _ _ _ _ _ _ _ _ _ _ _ _ _ _ _ _ _ _ _ _ _ _ _ _ _ _ _ _ _ _ _]
          tunnel: w134 -> [w165 w177 w182 w191 w214 w222 w239 w261 w281 w291 w304 w321 w327 w333 w342 w354 w361 w373 w387 w399 w432 w434 w442 w460 w479 w496 w514 w527 w537 w541 w543 w561 w567 w584 w597 w610 w623 w647 w648 w669 w680 w693 w709 w717 w727 w746 w755 w776 w784 w789]
          tunnel: [w161 w177 w182 w184 w211 w220 w230 w255 w279 w290 w306 w320 w326 w332 w347 w349 w359 w376 w388 w404 w417 w433 w440 w458 w478 w489 w510 w527 w537 w540 w542 w557 w565 w583 w596 w609 w622 w639 w649 w656 w679 w697 w708 w715 w723 w740 w752 w776 w784 w789] -> w147
          tunnel: w133 -> [_ _ _ _ _ _ w226 _ _ _ _ _ _ _ _ _ _ _ _ _ _ _ _ _ _ _ _ w528 _ _ _ _ _ _ _ _ _ _ _ _ _ _ _ _ _ _ _ w777 _ _]
          event "OK": Value Change {
            n80 = event-data() -> ()  [unwired: 2 out]
            n81 = call "Finalize Text.vi"("error in (no error)"=w168, "Data in"=w165) -> ("error out"=w169:errorcluster, "Data out"=w164:T28)  [unwired: 8 out]
            n82 = call "Finalize Movement.vi"("error in (no error)"=w169, "Data in"=w164) -> ("error out"=w170:errorcluster, "Data out"=w163:T28)  [unwired: 1 in, 7 out]
            n83 = call "DeselectLayer.vi"("error in (no error)"=w170, "Data in"=w163) -> ("error out"=w167:errorcluster, "Data out"=w162:T28)  [unwired: 8 out]
            n84 = call "Reset layer template selection.vi"("error in (no error)"=w167, "Data in"=w162) -> ("error out"=w166:errorcluster, "Data out"=w161:T28)  [unwired: 1 in, 7 out]
          }
          event "Cancel": Value Change {
            n85 = event-data() -> ()  [unwired: 2 out]
            n86 = control-ref of="This VI"() -> (w173:refnum<vi>)
            n87 = call "Verify Cancel.vi"("Calling VI"=w173) -> ("error out"=w176:errorcluster, "Close IE"=w175:bool)  [unwired: 9 in]
          }
          event Panel Close? {
            w179 = TRUE ("Discard?")
            n88 = event-data() -> ()  [unwired: 2 out]
            n89 = control-ref of="This VI"() -> (w178:refnum<vi>)
            n90 = call "Verify Cancel.vi"("Calling VI"=w178) -> ("error out"=w181:errorcluster, "Close IE"=w180:bool)  [unwired: 9 in]
            n91 = event-data("Discard?"=w179) -> ()  [unwired: 1 in, 1 out]
          }
          event Mouse Up {
            # "Has check for anything changing"
            n92 = event-data() -> ()  [unwired: 2 out]
            n93 = Unbundle By Name(w191) -> ("Support.Action"=w189:T32, "Support.Mouse inside icon?"=w194:bool, "Support.Mouse Move Coords"=w190:T31)
            n94 = case shown="False" w194 {
              tunnel: w192 -> [w198 w209]
              tunnel: [w196 w209] -> w187
              tunnel: [w199 w208] -> w185
              tunnel: w191 -> [w200 w208]
              tunnel: w190 -> [w197 _]
              tunnel: w189 -> [w195 _]
              frame False {
                n95 = case shown="\"Move Selection\", \"Tool\"" w195 {
                  tunnel: w200 -> [w202 w207]
                  tunnel: [w202 w206] -> w199
                  tunnel: w198 -> [w201 w205]
                  tunnel: w197 -> [_ w204]
                  tunnel: [w201 w203] -> w196
                  frame "Default", Default {
                  }
                  frame "Move Selection", "Tool" {
                    n96 = call "PictureControl_MouseUp.vi"("error in"=w205, "Coords"=w204, "Data in"=w207) -> ("error out"=w203:errorcluster, "Data out"=w206:T28)  [unwired: 4 in, 3 out]
                  }
                }
              }
              frame True {
              }
            }
            n97 = call "Add Data to History.vi"("Check special fields? (F)"=TRUE, "Add to Undo?"=TRUE, "error in"=w187, "Data in"=w185) -> ("error out"=w186:errorcluster, "Data out"=w184:T28)  [unwired: 6 out]
          }
          event Key Down?; event type 5.0.x8000000b {
            n98 = event-data() -> ("Type"=w213:T35, "Char"=w210:i16, "VKey"=w217:T36, "PlatMods"=w212:T37)  [unwired: 1 out]
            n99 = call "KeyDown.vi"("PlatMods"=w212, "Type"=w213, "error in (no error)"=w219, "VKey"=w217, "Char"=w210, "Data in"=w214) -> ("error out"=w218:errorcluster, "Discard?"=w216:bool, "Data out"=w211:T28)  [unwired: 3 out]
            n100 = event-data("Discard?"=w216) -> ()  [unwired: 1 in, 1 out]
          }
          event Key Up {
            n101 = event-data() -> ("PlatMods"=w221:T37)  [unwired: 1 out]
            n102 = call "KeyUp.vi"("error in (no error)"=w223, "PlatMods"=w221, "Data in"=w222) -> ("error out"=w224:errorcluster, "Data out"=w220:T28)  [unwired: 7 out]
          }
          event Menu Selection (User); Menu Selection (App) {
            n103 = event-data() -> ("Type"=w237:T35, "ItemTag"=w238:string)  [unwired: 1 out]
            n104 = case shown="\"Text\"" w234 {
              tunnel: w236 -> [w240 w245]
              tunnel: w239 -> [w241 w244]
              tunnel: [w240 w243] -> w232
              tunnel: [w241 w242] -> w233
              frame Default {
              }
              frame "Text" {
                n105 = call "Finalize Text.vi"("error in (no error)"=w245, "Data in"=w244) -> ("error out"=w243:errorcluster, "Data out"=w242:T28)  [unwired: 8 out]
              }
            }
            n106 = control-ref of="Clipboard"() -> (w225:refnum<vi>)
            n107 = case shown="\"Menu Selection (User)\"" w237 {
              tunnel: w238 -> [_ w254]
              tunnel: [w247 w253] -> w229
              tunnel: w232 -> [w247 w252]
              tunnel: w226 -> [_ w251]
              tunnel: w233 -> [w246 w250]
              tunnel: [w246 w249] -> w231
              tunnel: w225 -> [_ w248]
              frame Default {
              }
              frame "Menu Selection (User)" {
                n108 = call "MenuSelection(User).vi"("User events"=w251, "Clipboard"=w248, "error in"=w252, "ItemTag"=w254, "Data in"=w250) -> ("error out"=w253:errorcluster, "Data out"=w249:T28)  [unwired: 5 out]
              }
            }
            n109 = call "Add Data to History.vi"("Add to Undo?"=FALSE, "error in"=w229, "Data in"=w231) -> ("error out"=w228:errorcluster, "Data out"=w230:T28)  [unwired: 7 in]
          }
          event "Tab Control": Value Change {
            n110 = event-data() -> ("NewVal"=w266:T3)  [unwired: 1 out]
            n111 = case shown="\"Layers\", Default" w266 {
              tunnel: w265 -> [w270 w273 w275 w277]
              tunnel: [w269 w272 w276 w277] -> w264
              frame "Templates" {
                n112 = property on="Filter templates by keyword" class="Str"(error in=w270, "Key Focus"=TRUE) -> (error out=w269:errorcluster)  [unwired: 1 in, 1 out]
              }
              frame "Glyphs" {
                n113 = property on="Filter glyphs by keyword" class="Str"(error in=w273, "Key Focus"=TRUE) -> (error out=w272:errorcluster)  [unwired: 1 in, 1 out]
              }
              frame "Icon Text" {
                n114 = property on="Line 1 text" class="Str"(error in=w275, "Key Focus"=TRUE) -> (error out=w276:errorcluster)  [unwired: 1 in, 1 out]
              }
              frame "Layers", Default {
              }
            }
            n115 = call "Finalize Text.vi"("error in (no error)"=w264, "Data in"=w261) -> ("error out"=w267:errorcluster, "Data out"=w260:T28)  [unwired: 8 out]
            n116 = call "Finalize Movement.vi"("error in (no error)"=w267, "Data in"=w260) -> ("error out"=w259:errorcluster, "Data out"=w257:T28)  [unwired: 1 in, 7 out]
            n117 = call "Escape.vi"("error in"=w259, "Data in"=w257) -> ("error out"=w258:errorcluster, "Data out"=w256:T28)  [unwired: 1 in, 7 out]
            n118 = call "Reset layer template selection.vi"("error in (no error)"=w258, "Data in"=w256) -> ("error out"=w263:errorcluster, "Data out"=w255:T28)  [unwired: 1 in, 7 out]
          }
          event "Preview", "Terminals", "Preview2": Mouse Enter {
            n119 = event-data() -> ()  [unwired: 2 out]
            n120 = call "SetCursor.vi"("error in (no error)"=w285, "Radio Buttons"=w283, "Data in"=w281) -> ("error out"=w284:errorcluster, "Data out"=w280:T28)  [unwired: 7 out]
            n121 = Bundle By Name(cluster=w280, "Support.Mouse inside icon?"=TRUE) -> (w279:T28)
          }
          event "Preview", "Terminals", "Preview2": Mouse Move {
            n122 = event-data() -> ("Coords"=w289:T31)  [unwired: 1 out]
            n123 = call "CoordinatesCorrection.vi"("Coordinates In"=w289) -> ("Corrected Out"=w286:T31)  [unwired: 10 out]
            n124 = feedback-in #1(w286) -> ()
            n125 = feedback #1() -> (w288:T31)
            n126 = Not Equal?(x=w288, y=w286) -> (x != y?=w287:bool)
            n127 = case shown="True" w287 {
              tunnel: w295 -> [w297 w303]
              tunnel: [w297 w302] -> w294
              tunnel: w292 -> [_ w301]
              tunnel: w291 -> [w296 w300]
              tunnel: [w296 w299] -> w290
              tunnel: w286 -> [_ w298]
              frame False {
              }
              frame True {
                n128 = call "MouseMove.vi"("Buffer"=w301, "error in"=w303, "Coords"=w298, "Data in"=w300) -> ("error out"=w302:errorcluster, "Data out"=w299:T28)  [unwired: 6 out]
              }
            }
          }
          event "Preview", "Preview2", "Terminals": Mouse Leave {
            n129 = event-data() -> ()  [unwired: 2 out]
            n130 = Bundle By Name(cluster=w304, "Support.Mouse inside icon?"=FALSE) -> (w306:T28)
          }
          event "Preview", "Terminals", "Preview2": Mouse Down {
            # "Left click"
            n131 = event-data() -> ("Button"=w310:u16, "Coords"=w323:T31)  [unwired: 1 out]
            n132 = Not Equal?(x=u16 1, y=w310) -> (x != y?=w308:bool)
            n133 = control-ref of="This VI"() -> (w319:refnum<vi>)
            n134 = call "Defer_FP_Updates.vi"("Defer Panel Updates"=TRUE, "error in"=w325, "lv_icon.vi in"=w319) -> ("error out"=w315:errorcluster, "lv icon.vi out"=w317:refnum<vi>)  [unwired: 7 out]
            n135 = call "Reset layer template selection.vi"("Force reset? (T)"=FALSE, "error in (no error)"=w315, "Data in"=w321) -> ("error out"=w314:errorcluster, "Data out"=w311:T28)  [unwired: 1 in, 6 out]
            n136 = call "MouseDown.vi"("Flip colors?"=w308, "error in"=w314, "Coords"=w323, "Data in"=w311) -> ("error out"=w313:errorcluster, "Data out"=w320:T28)  [unwired: 1 in, 5 out]
            n137 = call "Defer_FP_Updates.vi"("Defer Panel Updates"=FALSE, "error in"=w313, "lv_icon.vi in"=w317) -> ("error out"=w324:errorcluster)  [unwired: 8 out]
          }
          event "Preview", "Terminals", "Preview2": Mouse Up {
            n138 = event-data() -> ("Coords"=w330:T31)  [unwired: 1 out]
            n139 = call "PictureControl_MouseUp.vi"("error in"=w331, "Coords"=w330, "Data in"=w327) -> ("error out"=w328:errorcluster, "Data out"=w326:T28)  [unwired: 4 in, 3 out]
          }
          event Value Change {
            n140 = event-data() -> ("NewVal"=w335:T20)  [unwired: 1 out]
            n141 = call "Value Change_Tools.vi"("error in"=w336, "NewVal"=w335, "Data in"=w333) -> ("error out"=w334:errorcluster, "Data out"=w332:T28)  [unwired: 7 out]
          }
          event Mouse Down {
            n142 = event-data() -> ("Mods.Double Click"=w337:bool)  [unwired: 1 out]
            n143 = call "Finalize Text.vi"("error in (no error)"=w343, "Data in"=w342) -> ("error out"=w345:errorcluster, "Data out"=w344:T28)  [unwired: 8 out]
            n144 = call "Finalize Movement.vi"("error in (no error)"=w345, "Data in"=w344) -> ("error out"=w341:errorcluster, "Data out"=w340:T28)  [unwired: 1 in, 7 out]
            n145 = call "Mouse Down.vi"("error in"=w341, "Double Click"=w337, "Data in"=w340) -> ("error out"=w338:errorcluster, "Data out"=w339:T28)  [unwired: 7 out]
            n146 = Bundle By Name(cluster=w339, "Support.Tool (old value)"=u32 111) -> (w347:T28)
          }
          event Mouse Down {
            n147 = event-data() -> ()  [unwired: 2 out]
            n148 = call "Finalize Text.vi"("error in (no error)"=w355, "Data in"=w354) -> ("error out"=w356:errorcluster, "Data out"=w353:T28)  [unwired: 8 out]
            n149 = call "Finalize Movement.vi"("error in (no error)"=w356, "Data in"=w353) -> ("error out"=w352:errorcluster, "Data out"=w350:T28)  [unwired: 1 in, 7 out]
            n150 = call "Escape.vi"("error in"=w352, "Data in"=w350) -> ("error out"=w351:errorcluster, "Data out"=w349:T28)  [unwired: 1 in, 7 out]
          }
          event Value Change {
            n151 = event-data() -> ()  [unwired: 2 out]
            n152 = call "Check Color.vi"("Color in"="Fill Color") -> ("Color out"=w364:T19)  [unwired: 26 out]
            n153 = call "Check Color.vi"("Color in"="Line Color") -> ("Color out"=w365:T19)  [unwired: 26 out]
            n154 = Bundle By Name(cluster=w361, "Support.Fill Color"=w364, "Support.Edge Color"=w365) -> (w360:T28)
            n155 = call "Escape.vi"("Reset cursor (T)"=FALSE ("Reset cursor? (T)"), "error in"=w362, "Data in"=w360) -> ("error out"=w363:errorcluster, "Data out"=w359:T28)  [unwired: 1 in, 6 out]
          }
          event Value Change {
            n156 = event-data() -> ()  [unwired: 2 out]
            n157 = call "Finalize Text.vi"("error in (no error)"=w371, "Data in"=w373) -> ("error out"=w375:errorcluster, "Data out"=w374:T28)  [unwired: 8 out]
            n158 = local read "Line Color"() -> (w370:T19)
            n159 = local read "Fill Color"() -> (w380:T19)
            n160 = call "Finalize Movement.vi"("error in (no error)"=w375, "Data in"=w374) -> ("error out"=w369:errorcluster, "Data out"=w372:T28)  [unwired: 1 in, 7 out]
            n161 = stacked-sequence {
              tunnel: w380 -> [w384]
              tunnel: [w383] -> w378
              tunnel: w370 -> [w382]
              tunnel: w369 -> [w381]
              frame #0 {
                n162 = local write "Fill Color"(w382) -> ()
                n163 = property on="Line Color" class="ColBox (strict)"(error in=w381, "Val(Sgnl)"=w384) -> (error out=w383:errorcluster)  [unwired: 1 in, 1 out]
              }
            }
            n164 = call "Escape.vi"("error in"=w378, "Data in"=w372) -> ("error out"=w377:errorcluster, "Data out"=w376:T28)  [unwired: 1 in, 7 out]
          }
          event Value Change {
            n165 = event-data() -> ()  [unwired: 2 out]
            n166 = call "Finalize Text.vi"("error in (no error)"=w394, "Data in"=w387) -> ("error out"=w393:errorcluster, "Data out"=w389:T28)  [unwired: 8 out]
            n167 = call "Finalize Movement.vi"("error in (no error)"=w393, "Data in"=w389) -> ("error out"=w390:errorcluster, "Data out"=w386:T28)  [unwired: 1 in, 7 out]
            n168 = call "RotateFlip.vi"("error in"=w390, "Rotate"="Clockwise Rotate", "Data in"=w386) -> ("error out"=w391:errorcluster, "Data out"=w385:T28)  [unwired: 2 in, 5 out]
            n169 = call "Escape.vi"("error in"=w391, "Data in"=w385) -> ("error out"=w392:errorcluster, "Data out"=w388:T28)  [unwired: 1 in, 7 out]
          }
          event User Event {
            # "This is an initialization event for the templates"
            n170 = event-data() -> ("Templates"=w414:string)  [unwired: 1 out]
            n171 = Unbundle By Name(w399) -> ("Ref.TemplateLoadAnimation"=w398:refnum<vi>, "Ref.refreshTemplates"=w397:refnum<vi>)
            n172 = control-ref of="This VI"() -> (w409:refnum<vi>)
            n173 = call "Defer_FP_Updates.vi"("Defer Panel Updates"=TRUE, "error in"=w412, "lv_icon.vi in"=w409) -> ("error out"=w407:errorcluster, "lv icon.vi out"=w406:refnum<vi>)  [unwired: 7 out]
            n174 = Unflatten From String(type=cluster{T6[], i32, bool} {[], 0, FALSE}, binary string=w414, error in (no error)=w407) -> (value=w405:cluster{T6[], i32, bool}, error out=w410:errorcluster)  [unwired: 3 out]
            n175 = call "Process Template Graphics.vi"("error in (no error)"=w410, "Data"=w405, "Data in"=w399) -> ("error out"=w402:errorcluster, "Data out"=w404:T28)  [unwired: 7 out]
            n176 = call "ChangeRefreshGraphicsState.vi"("error in (no error)"=w402, "refreshing?"=FALSE, "button ref"=w397, "animatedDecoration ref"=w398) -> ("error out"=w401:errorcluster)  [unwired: 7 in]
            n177 = call "Defer_FP_Updates.vi"("error in"=w401, "lv_icon.vi in"=w406) -> ("error out"=w403:errorcluster)  [unwired: 1 in, 8 out]
          }
          event "Templates": Value Change {
            n178 = event-data() -> ("CtlRef"=w416:refnum<vi>, "NewVal"=w427:string)  [unwired: 1 out]
            n179 = control-ref of="This VI"() -> (w431:refnum<vi>)
            n180 = Unbundle By Name(w432) -> ("Class.Templates"=w419:refnum<class "FakedArray.lvclass">)
            n181 = call "Defer_FP_Updates.vi"("Defer Panel Updates"=TRUE, "error in"=w429, "lv_icon.vi in"=w431) -> ("error out"=w421:errorcluster, "lv icon.vi out"=w426:refnum<vi>)  [unwired: 7 out]
            n182 = call-dynamic "SET_ScrollbarPosition.vi"("error in (no error)"=w421, "FakedArray.lvclass in"=w419) -> ("error out"=w423:errorcluster, "FakedArray.lvclass out"=w422:refnum<class "FakedArray.lvclass">)  [unwired: 1 in, 7 out]
            n183 = local write "Filter templates by keyword"("") -> ()
            n184 = call "ResetColor.vi"("error in (no error)"=w423, "FakedArray in"=w422) -> ("error out"=w424:errorcluster, "FakedArray out"=w425:refnum<class "FakedArray.lvclass">)  [unwired: 8 out]
            n185 = call-dynamic "UpdateVisibleData.vi"("Templates tree"=w416, "error in (no error)"=w424, "Tag"=w427, "FakedArray in"=w425) -> ("error out"=w420:errorcluster, "FakedArray out"=w418:refnum<class "FakedArray.lvclass">)  [unwired: 1 in, 5 out]
            n186 = Bundle By Name(cluster=w432, "Class.Templates"=w418) -> (w417:T28)
            n187 = call "Defer_FP_Updates.vi"("error in"=w420, "lv_icon.vi in"=w426) -> ("error out"=w428:errorcluster)  [unwired: 1 in, 8 out]
          }
          event "Templates": Mouse Down {
            n188 = event-data() -> ("CtlRef"=w437:refnum<vi>, "Coords"=w439:T31)  [unwired: 1 out]
            n189 = call "Mouse Down_Tree.vi"("Tree"=w437, "error in (no error)"=w438, "Coords"=w439) -> ("error out"=w436:errorcluster)  [unwired: 8 out]
            n190 = call "Escape.vi"("error in"=w436, "Data in"=w434) -> ("error out"=w435:errorcluster, "Data out"=w433:T28)  [unwired: 1 in, 7 out]
          }
          event Value Change {
            n191 = event-data() -> ("OldVal.Opacity"=w444:u8, "NewVal.Opacity"=w445:u8, "NewVal"=w449:T14)  [unwired: 1 out]
            n192 = Not Equal?(x=w444, y=w445) -> (x != y?=w443:bool)
            n193 = call "Value Change_Top or Bottom Layer.vi"("Type"=enum16{"Template Layer", "Text Layer"}."Template Layer", "error in (no error)"=w451, "Data"=w449, "Data in"=w442) -> ("error out"=w447:errorcluster, "Data out"=w441:T28)  [unwired: 6 out]
            n194 = case shown="False" w443 {
              tunnel: w447 -> [w453 w457]
              tunnel: [w453 w456] -> w446
              tunnel: w441 -> [w452 w455]
              tunnel: [w452 w454] -> w440
              frame False {
              }
              frame True {
                n195 = call "Reset layer template selection.vi"("error in (no error)"=w457, "Data in"=w455) -> ("error out"=w456:errorcluster, "Data out"=w454:T28)  [unwired: 1 in, 7 out]
              }
            }
          }
          event Mouse Down {
            n196 = event-data() -> ("CtlRef"=w463:refnum<vi>, "Button"=w459:u16)  [unwired: 1 out]
            n197 = case shown="1, 2" w459 {
              tunnel: w464 -> [w466 w473]
              tunnel: w463 -> [_ w477]
              tunnel: [w466 w471] -> w462
              tunnel: w460 -> [w465 w468]
              tunnel: [w465 w467] -> w458
              frame 0, Default {
              }
              frame 1, 2 {
                n198 = control-ref of="This VI"() -> (w476:refnum<vi>)
                n199 = call "Defer_FP_Updates.vi"("Defer Panel Updates"=TRUE, "error in"=w473, "lv_icon.vi in"=w476) -> ("error out"=w474:errorcluster, "lv icon.vi out"=w469:refnum<vi>)  [unwired: 7 out]
                n200 = call "Template_MouseDown.vi"("Add to Undo?"=TRUE, "error in"=w474, "CtlRef"=w477, "Data in"=w468) -> ("error out"=w472:errorcluster, "Data out"=w467:T28)  [unwired: 1 in, 5 out]
                n201 = call "Defer_FP_Updates.vi"("error in"=w472, "lv_icon.vi in"=w469) -> ("error out"=w471:errorcluster)  [unwired: 1 in, 8 out]
              }
            }
          }
          event Value Change {
            n202 = event-data() -> ("NewVal"=w488:variant)  [unwired: 1 out]
            n203 = control-ref of="This VI"() -> (w485:refnum<vi>)
            n204 = call "Defer_FP_Updates.vi"("Defer Panel Updates"=TRUE, "error in"=w486, "lv_icon.vi in"=w485) -> ("error out"=w487:errorcluster, "lv icon.vi out"=w480:refnum<vi>)  [unwired: 7 out]
            n205 = call "Mouse Down_Templates.vi"("Tag"="Templates", "error in"=w487, "NewVal"=w488, "Data in"=w479) -> ("error out"=w482:errorcluster, "Data out"=w478:T28)  [unwired: 1 in, 5 out]
            n206 = call "Defer_FP_Updates.vi"("error in"=w482, "lv_icon.vi in"=w480) -> ("error out"=w483:errorcluster)  [unwired: 1 in, 8 out]
          }
          event "Filter templates by keyword": Value Change {
            n207 = event-data() -> ("NewVal"=w508:string)  [unwired: 1 out]
            n208 = Unbundle By Name(w496) -> ("Ref.Templates tree"=w494:refnum<vi>, "Class.Templates"=w497:refnum<class "FakedArray.lvclass">)
            n209 = control-ref of="This VI"() -> (w507:refnum<vi>)
            n210 = call "Defer_FP_Updates.vi"("Defer Panel Updates"=TRUE, "error in"=w505, "lv_icon.vi in"=w507) -> ("error out"=w499:errorcluster, "lv icon.vi out"=w504:refnum<vi>)  [unwired: 7 out]
            n211 = call-dynamic "SET_ScrollbarPosition.vi"("error in (no error)"=w499, "FakedArray.lvclass in"=w497) -> ("error out"=w500:errorcluster, "FakedArray.lvclass out"=w501:refnum<class "FakedArray.lvclass">)  [unwired: 1 in, 7 out]
            n212 = call "ResetColor.vi"("error in (no error)"=w500, "FakedArray in"=w501) -> ("error out"=w502:errorcluster, "FakedArray out"=w503:refnum<class "FakedArray.lvclass">)  [unwired: 8 out]
            n213 = call-dynamic "UpdateVisibleData.vi"("Templates tree"=w494, "error in (no error)"=w502, "Keyword"=w508, "FakedArray in"=w503) -> ("error out"=w498:errorcluster, "FakedArray out"=w495:refnum<class "FakedArray.lvclass">)  [unwired: 1 in, 5 out]
            n214 = Bundle By Name(cluster=w496, "Class.Templates"=w495) -> (w490:T28)
            n215 = call "Defer_FP_Updates.vi"("error in"=w498, "lv_icon.vi in"=w504) -> ("error out"=w492:errorcluster)  [unwired: 1 in, 8 out]
            n216 = call "Add Data to History.vi"("Add to Undo?"=TRUE, "error in"=w492, "Data in"=w490) -> ("error out"=w491:errorcluster, "Data out"=w489:T28)  [unwired: 7 out]
          }
          event "Filter templates by keyword": Mouse Down {
            # "If a mouse down event should\nselect the entered text, enable this case"
            n217 = event-data() -> ("CtlRef"=w518:refnum<vi>)  [unwired: 1 out]
            n218 = disable-structure shown="Enabled" {
              disable-tunnel: w518 -> [w523 _]
              disable-tunnel: w517 -> [w521 w524]
              disable-tunnel: [w519 w524] -> w516
              frame Disabled {
                n219 = property class="Str"(reference=w523, error in=w521, "Text.Selection Start"=u32 0 ("Text.Selection:Start"), "Text.Selection End"=-1 ("Text.Selection:End")) -> (error out=w519:errorcluster)  [unwired: 1 out]
              }
              frame Enabled {
              }
            }
            n220 = call "Finalize Text.vi"("error in (no error)"=w516, "Data in"=w514) -> ("error out"=w515:errorcluster, "Data out"=w513:T28)  [unwired: 8 out]
            n221 = call "DeselectLayer.vi"("error in (no error)"=w515, "Data in"=w513) -> ("error out"=w512:errorcluster, "Data out"=w511:T28)  [unwired: 8 out]
            n222 = call "Escape.vi"("error in"=w512, "Data in"=w511) -> ("error out"=w509:errorcluster, "Data out"=w510:T28)  [unwired: 1 in, 7 out]
          }
          event Value Change {
            n223 = event-data() -> ()  [unwired: 2 out]
            n224 = Unbundle By Name(w527) -> ("Ref.TemplateLoadAnimation"=w525:refnum<vi>, "Ref.refreshTemplates"=w526:refnum<vi>)
            n225 = call "Launch Dynamically Load Graphics.vi"("User events"=w528, "Path"=Pathes."Icon Templates", "error in (no error)"=w530, "button ref"=w526, "animatedDecoration ref"=w525) -> ("error out"=w529:errorcluster)  [unwired: 1 in, 5 out]
          }
          event Mouse Down {
            n226 = event-data() -> ("CtlRef"=w536:refnum<vi>)  [unwired: 1 out]
            n227 = property class="CmbBox (strict)"(reference=w536, error in=w535, "Text.Selection Start"=u32 0 ("Text.Selection:Start"), "Text.Selection End"=u32 1000 ("Text.Selection:End")) -> (error out=w534:errorcluster)  [unwired: 1 out]
          }
          event Mouse Down {
            n228 = event-data() -> ()  [unwired: 2 out]
            n229 = call "Escape.vi"("error in"=w539, "Data in"=w541) -> ("error out"=w538:errorcluster, "Data out"=w540:T28)  [unwired: 1 in, 7 out]
          }
          event Mouse Down {
            n230 = event-data() -> ()  [unwired: 2 out]
            n231 = call "MouseDown_Body Text.vi"("error in"=w546, "Data in"=w543) -> ("error out"=w545:errorcluster, "Data out"=w542:T28)  [unwired: 8 out]
          }
          event Value Change {
            n232 = event-data() -> ("OldVal"=w555:T7, "NewVal"=w554:T7, "OldVal.Body Text Spec.Alignment"=w559:T9)  [unwired: 1 out]
            n233 = Unbundle By Name(w555) -> ("Body Text Spec.Font"=w553:T8)
            n234 = Unbundle By Name(w554) -> ("Body Text Spec.Font"=w552:T8)
            n235 = local read "Tab Control"() -> (w550:T3)
            n236 = Unbundle By Name(w554) -> ("Body Text Spec.Alignment"=w560:T9)
            n237 = Equal?(x=w550, y=T3."Icon Text") -> (x = y?=w548:bool)
            n238 = Not Equal?(x=w553, y=w552) -> (x != y?=w551:bool)
            n239 = And(x=w548, y=w551) -> (x .and. y?=w547:bool)
            n240 = Not Equal?(x=w560, y=w559) -> (x != y?=w558:bool)
            n241 = case shown="False" w547 {
              frame False {
              }
              frame True {
                n242 = property on="Line 1 text" class="Str"("Key Focus"=TRUE) -> ()  [unwired: 2 in, 2 out]
              }
            }
            n243 = call "Alignment Value Change.vi"("Set Focus?"=w558, "error in"=w563, "NewVal"=w560, "Data in"=w561) -> ("error out"=w556:errorcluster, "Data out"=w557:T28)  [unwired: 6 out]
          }
          event Value Change {
            n244 = event-data() -> ("OldVal.Opacity"=w570:u8, "NewVal.Opacity"=w569:u8, "NewVal"=w575:T14)  [unwired: 1 out]
            n245 = Not Equal?(x=w570, y=w569) -> (x != y?=w568:bool)
            n246 = call "Value Change_Top or Bottom Layer.vi"("Type"=enum16{"Template Layer", "Text Layer"}."Text Layer", "error in (no error)"=w576, "Data"=w575, "Data in"=w567) -> ("error out"=w572:errorcluster, "Data out"=w566:T28)  [unwired: 6 out]
            n247 = case shown="True" w568 {
              tunnel: w572 -> [w578 w582]
              tunnel: [w578 w581] -> w571
              tunnel: w566 -> [w577 w580]
              tunnel: [w577 w579] -> w565
              frame False {
              }
              frame True {
                n248 = call "Reset layer template selection.vi"("error in (no error)"=w582, "Data in"=w580) -> ("error out"=w581:errorcluster, "Data out"=w579:T28)  [unwired: 1 in, 7 out]
              }
            }
          }
          event Value Change {
            n249 = event-data() -> ("NewVal"=w593:variant)  [unwired: 1 out]
            n250 = control-ref of="This VI"() -> (w590:refnum<vi>)
            n251 = call "Defer_FP_Updates.vi"("Defer Panel Updates"=TRUE, "error in"=w589, "lv_icon.vi in"=w590) -> ("error out"=w588:errorcluster, "lv icon.vi out"=w585:refnum<vi>)  [unwired: 7 out]
            n252 = Variant To Data(error in=w588, type=0, Variant=w593) -> (data=w592:i32, error out=w594:errorcluster)
            n253 = call "UpdateLayerView_ScrollbarChanged.vi"("error in"=w594, "Scrollbar Position"=w592, "Data in"=w584) -> ("error out"=w587:errorcluster, "Data out"=w583:T28)  [unwired: 7 out]
            n254 = call "Defer_FP_Updates.vi"("error in"=w587, "lv_icon.vi in"=w585) -> ("error out"=w586:errorcluster)  [unwired: 1 in, 8 out]
          }
          event Mouse Down {
            n255 = event-data() -> ("PlatMods.Shift"=w598:bool, "CtlRef"=w608:refnum<vi>, "PlatMods.Ctrl"=w607:bool)  [unwired: 1 out]
            n256 = control-ref of="This VI"() -> (w604:refnum<vi>)
            n257 = call "Defer_FP_Updates.vi"("Defer Panel Updates"=TRUE, "error in"=w605, "lv_icon.vi in"=w604) -> ("error out"=w603:errorcluster, "lv icon.vi out"=w600:refnum<vi>)  [unwired: 7 out]
            n258 = call "Mouse Down_User Layers.vi"("Shift"=w598, "error in"=w603, "Ctrl"=w607, "CtlRef"=w608, "Data in"=w597) -> ("error out"=w602:errorcluster, "Data out"=w596:T28)  [unwired: 5 out]
            n259 = call "Defer_FP_Updates.vi"("error in"=w602, "lv_icon.vi in"=w600) -> ("error out"=w601:errorcluster)  [unwired: 1 in, 8 out]
          }
          event Mouse Down {
            n260 = event-data() -> ("Button"=w611:u16)  [unwired: 1 out]
            n261 = case shown="1" w611 {
              tunnel: w613 -> [w615 w619]
              tunnel: [w615 w618] -> w612
              tunnel: w610 -> [w614 w617]
              tunnel: [w614 w616] -> w609
              frame 0, Default {
              }
              frame 1 {
                # "Left click"
                n262 = call "Reset layer template selection.vi"("error in (no error)"=w619, "Data in"=w617) -> ("error out"=w618:errorcluster, "Data out"=w616:T28)  [unwired: 1 in, 7 out]
              }
            }
          }
          event Value Change {
            # "We do not use the dynamic registerd event for Layer Clust.Value Change\nbecause it would be a huge effort to lock the front panel until this\nevent case has been completed."
            n263 = event-data() -> ("OldVal.Visibility?"=w621:bool, "CtlRef"=w635:refnum<vi>, "OldVal.LayerName"=w620:string)  [unwired: 1 out]
            n264 = control-ref of="This VI"() -> (w632:refnum<vi>)
            n265 = call "Defer_FP_Updates.vi"("Defer Panel Updates"=TRUE, "error in"=w631, "lv_icon.vi in"=w632) -> ("error out"=w630:errorcluster, "lv icon.vi out"=w627:refnum<vi>)  [unwired: 7 out]
            n266 = call "LayerCluster_ValueChange.vi"("Old Visibility?"=w621, "error in"=w630, "Old name"=w620, "CtlRef"=w635, "Data in"=w623) -> ("error out"=w629:errorcluster, "Data out"=w624:T28)  [unwired: 1 in, 4 out]
            n267 = call "Defer_FP_Updates.vi"("Defer Panel Updates"=FALSE, "error in"=w629, "lv_icon.vi in"=w627) -> ("error out"=w626:errorcluster)  [unwired: 8 out]
            n268 = call "Reset layer template selection.vi"("error in (no error)"=w626, "Data in"=w624) -> ("error out"=w625:errorcluster, "Data out"=w622:T28)  [unwired: 1 in, 7 out]
          }
          event Value Change {
            n269 = event-data() -> ()  [unwired: 2 out]
            n270 = control-ref of="This VI"() -> (w646:refnum<vi>)
            n271 = call "Defer_FP_Updates.vi"("Defer Panel Updates"=TRUE, "error in"=w645, "lv_icon.vi in"=w646) -> ("error out"=w643:errorcluster, "lv icon.vi out"=w642:refnum<vi>)  [unwired: 7 out]
            n272 = call "Add new Layer.vi"("error in"=w643, "Data in"=w647) -> ("error out"=w638:errorcluster, "Data out"=w640:T28)  [unwired: 8 out]
            n273 = call "ViewLayer.vi"("Add to Undo?"=TRUE, "error in (no error)"=w638, "Data in"=w640) -> ("error out"=w637:errorcluster, "Data out"=w639:T28)  [unwired: 1 in, 6 out]
            n274 = call "Defer_FP_Updates.vi"("error in"=w637, "lv_icon.vi in"=w642) -> ("error out"=w641:errorcluster)  [unwired: 1 in, 8 out]
          }
          event Mouse Leave; Mouse Up {
            n275 = event-data() -> ()  [unwired: 2 out]
            n276 = call "Add Data to History.vi"("Add to Undo?"=TRUE, "error in"=w651, "Data in"=w648) -> ("error out"=w650:errorcluster, "Data out"=w649:T28)  [unwired: 7 out]
          }
          event Value Change {
            n277 = event-data() -> ()  [unwired: 2 out]
            n278 = control-ref of="This VI"() -> (w663:refnum<vi>)
            n279 = Unbundle By Name(w669) -> ("Class.Icon"=w668:refnum<class "Icon.lvclass">)
            n280 = call "Defer_FP_Updates.vi"("Defer Panel Updates"=TRUE, "error in"=w662, "lv_icon.vi in"=w663) -> ("error out"=w661:errorcluster, "lv icon.vi out"=w653:refnum<vi>)  [unwired: 7 out]
            n281 = call-dynamic "GET_All User Layers.vi"("error in (no error)"=w661, "Icon.lvclass in"=w668) -> ("error out"=w675:errorcluster, "User Layer"=w671:refnum<class "Layer.lvclass">[], "Icon.lvclass out"=w670:refnum<class "Icon.lvclass">)  [unwired: 7 out]
            n282 = call "Delete Selected Layers.vi"("error in"=w675, "All Layers in"=w671, "Data in"=w669) -> ("error out"=w674:errorcluster, "All Layers out"=w672:refnum<class "Layer.lvclass">[], "Data out"=w666:T28)  [unwired: 6 in]
            n283 = call-dynamic "SET_UserLayers.vi"("error in (no error)"=w674, "Layers"=w672, "Icon.lvclass in"=w670) -> ("error out"=w673:errorcluster, "Icon.lvclass out"=w667:refnum<class "Icon.lvclass">)  [unwired: 7 in]
            n284 = Bundle By Name(cluster=w666, "Class.Icon"=w667) -> (w665:T28)
            n285 = call "Reset layer template selection.vi"("error in (no error)"=w673, "Data in"=w665) -> ("error out"=w655:errorcluster, "Data out"=w657:T28)  [unwired: 1 in, 7 out]
            n286 = call "ViewLayer.vi"("Add to Undo?"=TRUE, "error in (no error)"=w655, "Data in"=w657) -> ("error out"=w654:errorcluster, "Data out"=w656:T28)  [unwired: 2 in, 5 out]
            n287 = call "Defer_FP_Updates.vi"("error in"=w654, "lv_icon.vi in"=w653) -> ("error out"=w660:errorcluster)  [unwired: 1 in, 8 out]
          }
          event Value Change {
            n288 = event-data() -> ()  [unwired: 2 out]
            n289 = control-ref of="This VI"() -> (w686:refnum<vi>)
            n290 = call "Defer_FP_Updates.vi"("Defer Panel Updates"=TRUE, "error in"=w685, "lv_icon.vi in"=w686) -> ("error out"=w684:errorcluster, "lv icon.vi out"=w683:refnum<vi>)  [unwired: 7 out]
            n291 = call "MoveLayers.vi"("error in"=w684, "Arrow Up"="Move Up", "Data in"=w680) -> ("error out"=w676:errorcluster, "Data out"=w679:T28)  [unwired: 7 out]
            n292 = stacked-sequence {
              tunnel: [w689] -> w677
              tunnel: w676 -> [w689]
              frame #0 {
                w690 = FALSE ("Arrow Down")
                n293 = local write "Move Down"(w690) -> ()
                n294 = local write "Move Up"(w690) -> ()
              }
            }
            n295 = call "Defer_FP_Updates.vi"("Defer Panel Updates"=FALSE, "error in"=w677, "lv_icon.vi in"=w683) -> ("error out"=w682:errorcluster)  [unwired: 8 out]
          }
          event User Event {
            # "This is an initialization event for the glyphs."
            n296 = event-data() -> ("Glyphs"=w705:string)  [unwired: 1 out]
            n297 = Unbundle By Name(w693) -> ("Ref.GlyphLoadAnimation"=w692:refnum<vi>, "Ref.refreshGlyphs"=w691:refnum<vi>)
            n298 = Unflatten From String(type=T34[] [], binary string=w705, error in (no error)=w703) -> (value=w700:T34[], error out=w702:errorcluster)  [unwired: 3 out]
            n299 = call "Populate Graphics.vi"("error in"=w702, "Glyphs []"=w700, "Data in"=w693) -> ("error out"=w701:errorcluster, "Data out"=w697:T28)  [unwired: 7 out]
            n300 = call "Write Glyphs to  File.vi"("File Name"="Glyphs.bin", "Path"=Pathes."Glyphs", "error in (no error)"=w701, "Graphics []"=w700) -> ("error out"=w696:errorcluster)  [unwired: 7 out]
            n301 = call "ChangeRefreshGraphicsState.vi"("error in (no error)"=w696, "refreshing?"=FALSE, "button ref"=w691, "animatedDecoration ref"=w692) -> ("error out"=w695:errorcluster)  [unwired: 7 in]
          }
          event "Glyphs": Mouse Down {
            n302 = event-data() -> ("CtlRef"=w707:refnum<vi>, "Coords"=w712:T31)  [unwired: 1 out]
            n303 = local write "Filter glyphs by keyword"("") -> ()
            n304 = call "Mouse Down_Tree.vi"("Tree"=w707, "error in (no error)"=w713, "Coords"=w712) -> ("error out"=w711:errorcluster)  [unwired: 8 out]
            n305 = call "Escape.vi"("error in"=w711, "Data in"=w709) -> ("error out"=w710:errorcluster, "Data out"=w708:T28)  [unwired: 1 in, 7 out]
          }
          event "Glyphs": Value Change {
            n306 = event-data() -> ("NewVal"=w721:string)  [unwired: 1 out]
            n307 = Unbundle By Name(w717) -> ("Class.Glyph"=w718:refnum<class "Glyph.lvclass">, "Ref.DNL_Glyphs []"=w714:refnum<vi>)
            n308 = call "FilterGlyphs.vi"("error in (no error)"=w719, "DNL_Glyphs []"=w714, "Tag"=w721, "Glyph in"=w718) -> ("error out"=w720:errorcluster, "Glyph out"=w716:refnum<class "Glyph.lvclass">)  [unwired: 6 out]
            n309 = Bundle By Name(cluster=w717, "Class.Glyph"=w716) -> (w715:T28)
          }
          event "Filter glyphs by keyword": Mouse Down {
            # "If a mouse down event should\nselect the entered text, enable this case"
            n310 = event-data() -> ("CtlRef"=w730:refnum<vi>)  [unwired: 1 out]
            n311 = disable-structure shown="Disabled" {
              disable-tunnel: w731 -> [w734 w737]
              disable-tunnel: w730 -> [w733 _]
              disable-tunnel: [w732 w737] -> w729
              frame Disabled {
                n312 = property class="Str"(reference=w733, error in=w734, "Text.Selection Start"=u32 0 ("Text.Selection:Start"), "Text.Selection End"=-1 ("Text.Selection:End")) -> (error out=w732:errorcluster)  [unwired: 1 out]
              }
              frame Enabled {
              }
            }
            n313 = call "Finalize Text.vi"("error in (no error)"=w729, "Data in"=w727) -> ("error out"=w728:errorcluster, "Data out"=w726:T28)  [unwired: 8 out]
            n314 = call "DeselectLayer.vi"("error in (no error)"=w728, "Data in"=w726) -> ("error out"=w725:errorcluster, "Data out"=w724:T28)  [unwired: 8 out]
            n315 = call "Escape.vi"("error in"=w725, "Data in"=w724) -> ("error out"=w722:errorcluster, "Data out"=w723:T28)  [unwired: 1 in, 7 out]
          }
          event "Filter glyphs by keyword": Value Change {
            n316 = event-data() -> ("NewVal"=w751:string)  [unwired: 1 out]
            n317 = Unbundle By Name(w746) -> ("Class.Glyph"=w747:refnum<class "Glyph.lvclass">, "Ref.DNL_Glyphs []"=w744:refnum<vi>, "Ref.Glyphs tree"=w743:refnum<vi>)
            n318 = First Call?() -> (First Call?: T/F=w749:bool)
            n319 = Not(x=w749) -> (.not. x?=w750:bool)
            n320 = call "SearchGlyphs.vi"("Glyphs tree"=w743, "DNL_Glyphs []"=w744, "Reset position? (F)"=w750, "error in (no error)"=w748, "Keyword"=w751, "Glyph in"=w747) -> ("error out"=w742:errorcluster, "Glyph out"=w745:refnum<class "Glyph.lvclass">)  [unwired: 4 out]
            n321 = Bundle By Name(cluster=w746, "Class.Glyph"=w745) -> (w739:T28)
            n322 = call "Add Data to History.vi"("Add to Undo?"=TRUE, "error in"=w742, "Data in"=w739) -> ("error out"=w741:errorcluster, "Data out"=w740:T28)  [unwired: 7 out]
          }
          event "Glyphs []": Mouse Down {
            n323 = event-data() -> ("Button"=w760:u16, "Mods.Double Click"=w761:bool, "CtlRef"=w763:refnum<vi>, "Coords"=w764:T31)  [unwired: 1 out]
            n324 = case shown="1" w760 {
              tunnel: w764 -> [_ w773]
              tunnel: w763 -> [_ w772]
              tunnel: [w766 w771] -> w757
              tunnel: w762 -> [w766 w770]
              tunnel: w761 -> [_ w769]
              tunnel: w755 -> [w765 w768]
              tunnel: [w765 w767] -> w753
              frame 0, Default {
              }
              frame 1 {
                # "Left click"
                n325 = call "Mouse Down_Glyphs.vi"("Double Click"=w769, "Coords"=w773, "error in"=w770, "CtlRef"=w772, "Data in"=w768) -> ("error out"=w771:errorcluster, "Data out"=w767:T28)  [unwired: 1 in, 4 out]
              }
            }
            n326 = call "Reset layer template selection.vi"("error in (no error)"=w757, "Data in"=w753) -> ("error out"=w756:errorcluster, "Data out"=w754:T28)  [unwired: 1 in, 7 out]
            n327 = call "Update glyph path string.vi"("error in (no error)"=w756, "Data in"=w754) -> ("error out"=w758:errorcluster, "Data out"=w752:T28)  [unwired: 1 in, 7 out]
          }
          event Value Change {
            n328 = event-data() -> ()  [unwired: 2 out]
            n329 = Unbundle By Name(w776) -> ("Ref.GlyphLoadAnimation"=w774:refnum<vi>, "Ref.refreshGlyphs"=w775:refnum<vi>)
            n330 = call "Launch Dynamically Load Graphics.vi"("User events"=w777, "Path"=Pathes."Glyphs", "error in (no error)"=w779, "button ref"=w775, "animatedDecoration ref"=w774) -> ("error out"=w778:errorcluster)  [unwired: 1 in, 5 out]
          }
          event "Help": Value Change {
            n331 = event-data() -> ()  [unwired: 2 out]
            n332 = control-ref of="This VI"() -> (w783:refnum<vi>)
            n333 = property class="VI"(reference=w783) -> (error out=w781:errorcluster, "Help.URL"=w782:string)  [unwired: 1 in, 1 out]
            n334 = call "IE_Open Help Link.vi"("error in (no error)"=w781, "Help.URL"=w782) -> ()  [unwired: 9 in, 1 out]
          }
          event "Glyphs", "Templates": Item Close; "Glyphs", "Templates": event #0x1e {
            n335 = event-data() -> ("CtlRef"=w786:refnum<vi>)  [unwired: 1 out]
            n336 = call "DealWithScrollbars.vi"("error in (no error)"=w788, "Tree"=w786) -> ("error out"=w787:errorcluster)  [unwired: 9 in]
          }
        }
        n337 = case shown="True" w136 {
          tunnel: [_ w156] -> w139
          tunnel: w138 -> [w149 w153]
          tunnel: [w149 w158] -> w137
          tunnel: "Tools" -> [_ w157]
          tunnel: w147 -> [w148 w154]
          tunnel: [w148 w155] -> w146
          frame False {
          }
          frame True {
            n338 = call "Apply Body Text.vi"("error in"=w153, "Body Text"="Body Text", "Data in"=w154) -> ("error out"=w152:errorcluster, "Data out"=w150:T28)  [unwired: 2 in, 5 out]
            n339 = call "DrawIcon.vi"("Tools"=w157, "error in (no error)"=w152, "Data in"=w150) -> ("error out"=w158:errorcluster, "Icon"=w156:picture, "Data out"=w155:T28, "RGB"=→"RGB":string, "XYL"=→"XYZ":string)  [unwired: 2 in, 2 out]
            "Icon" <- w156
            "Preview" <- w156
          }
        }
        n340 = Or(x=w138, y=w143) -> (x .or. y?=w142:bool)
      }
      n341 = call "Buffer for lossless tracking.vi"("Ref Cluster"=w117, "User events"=w105, "error in (no error)"=w121, "Buffer"=w120) -> ()  [unwired: 8 out]
      n342 = call "Extract LV Icon Data.vi"("error in (no error)"=w111, "LabVIEW Icon in (original)"=w109, "Data in"=w113) -> ("error out"=w110:errorcluster, "LabVIEW Icon out"=w112:string, "Data out"=w108:T28)  [unwired: 6 in]
      n343 = call "Get Image Data.vi"("Pic In"=w128) -> ("image data out"=w116:T2)  [unwired: 2 in, 8 out]
      n344 = call "Get Image Data.vi"("depth (24)"=1 ("depth"), "Pic In"=w128) -> ("image data out"=w126:T2)  [unwired: 2 in, 7 out]
      n345 = call "SetCursor.vi"("Radio Buttons"=Tools."Select", "Data in"=w108) -> ("Data out"=w107:T28)  [unwired: 8 in, 1 out]
      n346 = Unbundle By Name(w110) -> ("code"=w129:i32)
      n347 = flat-sequence {
        tunnel: w132 -> [w791]
        tunnel: w130 -> [w799]
        tunnel: w110 -> [w798]
        tunnel: w105 -> [w796]
        tunnel: w107 -> [w792]
        frame #0 {
          # "Make sure the Keep IE in Memory VI runs and completes before the main Icon Editor panel is closed."
          n348 = Unbundle By Name(w796) -> ("Global stop?"=w795:refnum<user-event>, "Templates"=w794:refnum<user-event>, "Glyphs"=w793:refnum<user-event>)
          n349 = call "Write INI Tokens and VI Tags.vi"("error in"=w798, "Global Data in"=w792) -> ()  [unwired: 1 in, 9 out]
          n350 = Unregister For Events(event registration refnum=w791) -> ()  [unwired: 1 in, 1 out]
          n351 = Release Notifier(notifier=w799, force destroy? (F)=TRUE) -> ()  [unwired: 1 in, 3 out]
          n352 = global read "Data.vi" "Debug"() -> (w790:bool)
          n353 = Generate User Event(user event=w795, event data cluster=TRUE) -> ()  [unwired: 2 in, 2 out]
          n354 = Destroy User Event(user event=w794) -> ()  [unwired: 1 in, 1 out]
          n355 = Destroy User Event(user event=w793) -> ()  [unwired: 1 in, 1 out]
          n356 = case shown="False" w790 {
            frame False {
              n357 = call "Call Keep IE in Memory.vi"() -> ()  [unwired: 1 out]
            }
            frame True {
            }
          }
        }
        frame #1 {
          n358 = global read "Data.vi" "Debug"() -> (w801:bool)
          n359 = case shown="False" w801 {
            frame False {
              n360 = invoke class="VI" method="FP.Close"() -> ()  [unwired: 3 in, 3 out]
            }
            frame True {
            }
          }
        }
      }
      n361 = call-dynamic "GET_Notifier.vi"("error in (no error)"=w114, "Ants.lvclass in"=w118) -> ("error out"=w124:errorcluster, "Notifier"=w130:refnum<notifier>, "Ants.lvclass out"=w125:refnum<class "Ants.lvclass">)  [unwired: 7 out]
      n362 = call "RunningAnts.vi"("error in (no error)"=w124, "Ants in"=w125) -> ()  [unwired: 10 out]
    }
    frame Error {
      n363 = Unbundle By Name(w803) -> ("code"=w804:i32)
      n364 = call <vilib>:"Simple Error Handler.vi"("error in (no error)"=w803) -> ()  [unwired: 4 in, 5 out]
    }
  }
  "BW icon out" <- w69
  "Error code out" <- w73
  "Color icon out" <- w51
  "LabVIEW Icon out" <- w48
